vi "ORS_GalvoGenScanData3D_uw.vi"(0 "x_center":dbl, 1 "x_span":dbl=5.0, 2 "offset":dbl, 3 "span-factor":dbl=5.0, 4 "y_center":dbl, 5 "y_span":dbl=1.0, 6 "mode":i32=6, 7 "n_lines":i32=50, 8 "Custom trig.":T1={"n_frames to c. trig"=0, "custom trig length (frames)"=1, "n_frames between c. trig"=1, "n_custom trigger"=4}, 9 "n_frames same y pos":u32=4, 11 "flyback_lines":i32=4, 12 "galvo phase":i32, 13 "n_frames":i32=20, 16 "n_3D scans":u32=1 min=1, 17 "flyback frames":u16) -> (10 "t_data":dbl[](graph)=[5.0, 5.0, 5.0, 5.0, 5.0, 5.0, 5.0, 5.0, 5.0, 5.0, 5.0, 5.0, 5.0, 5.0, 5.0, 5.0, 5.0, 5.0, 5.0, 5.0, 5.0, 5.0, 5.0, 5.0, 5.0, 5.0, 5.0, 5.0, 5.0, 5.0, 5.0, 5.0, 5.0, 5.0, 5.0, 5.0, 5.0, 5.0, 5.0, 5.0, 5.0, 5.0, 5.0, 5.0, 5.0, 5.0, 5.0, 5.0, 5.0, 5.0, 0.0, 0.0, 0.0, 0.0, 5.0, 5.0, 5.0, 5.0, 5.0, 5.0, 5.0, 5.0, 5.0, 5.0, 5.0, 5.0, 5.0, 5.0, 5.0, 5.0, 5.0, 5.0, 5.0, 5.0, 5.0, 5.0, 5.0, 5.0, 5.0, 5.0, 5.0, 5.0, 5.0, 5.0, 5.0, 5.0, 5.0, 5.0, 5.0, 5.0, 5.0, 5.0, 5.0, 5.0, 5.0, 5.0, 5.0, 5.0, 5.0, 5.0, 5.0, 5.0, 5.0, 5.0, 0.0, 0.0, 0.0, 0.0, 5.0, 5.0, 5.0, 5.0, 5.0, 5.0, 5.0, 5.0, 5.0, 5.0, 5.0, 5.0, 5.0, 5.0, 5.0, 5.0, 5.0, 5.0, 5.0, 5.0, 5.0, 5.0, 5.0, 5.0, 5.0, 5.0, 5.0, 5.0, 5.0, 5.0, 5.0, 5.0, 5.0, 5.0, 5.0, 5.0, 5.0, 5.0, 5.0, 5.0, 5.0, 5.0, 5.0, 5.0, 5.0, 5.0, 5.0, 5.0, 5.0, 5.0, 0.0, 0.0, 0.0, 0.0, 5.0, 5.0, 5.0, 5.0, 5.0, 5.0, 5.0, 5.0, 5.0, 5.0, 5.0, 5.0, 5.0, 5.0, 5.0, 5.0, 5.0, 5.0, 5.0, 5.0, 5.0, 5.0, 5.0, 5.0, 5.0, 5.0, 5.0, 5.0, 5.0, 5.0, 5.0, 5.0, 5.0, 5.0, 5.0, 5.0, 5.0, 5.0, 5.0, 5.0, 5.0, 5.0, 5.0, 5.0, 5.0, 5.0, 5.0, 5.0, 5.0, 5.0, 0.0, 0.0, 0.0, 0.0, 5.0, 5.0, 5.0, 5.0, 5.0, 5.0, 5.0, 5.0, 5.0, 5.0, 5.0, 5.0, 5.0, 5.0, 5.0, 5.0, 5.0, 5.0, 5.0, 5.0, 5.0, 5.0, 5.0, 5.0, 5.0, 5.0, 5.0, 5.0, 5.0, 5.0, 5.0, 5.0, 5.0, 5.0, 5.0, 5.0, 5.0, 5.0, 5.0, 5.0, 5.0, 5.0, 5.0, 5.0, 5.0, 5.0, 5.0, 5.0, 5.0, 5.0, 0.0, 0.0, 0.0, 0.0, 5.0, 5.0, 5.0, 5.0, 5.0, 5.0, 5.0, 5.0, 5.0, 5.0, 5.0, 5.0, 5.0, 5.0, 5.0, 5.0, 5.0, 5.0, 5.0, 5.0, 5.0, 5.0, 5.0, 5.0, 5.0, 5.0, 5.0, 5.0, 5.0, 5.0, 5.0, 5.0, 5.0, 5.0, 5.0, 5.0, 5.0, 5.0, 5.0, 5.0, 5.0, 5.0, 5.0, 5.0, 5.0, 5.0, 5.0, 5.0, 5.0, 5.0, 0.0, 0.0, 0.0, 0.0, 5.0, 5.0, 5.0, 5.0, 5.0, 5.0, 5.0, 5.0, 5.0, 5.0, 5.0, 5.0, 5.0, 5.0, 5.0, 5.0, 5.0, 5.0, 5.0, 5.0, 5.0, 5.0, 5.0, 5.0, 5.0, 5.0, 5.0, 5.0, 5.0, 5.0, 5.0, 5.0, 5.0, 5.0, 5.0, 5.0, 5.0, 5.0, 5.0, 5.0, 5.0, 5.0, 5.0, 5.0, 5.0, 5.0, 5.0, 5.0, 5.0, 5.0, 0.0, 0.0, 0.0, 0.0, 5.0, 5.0, 5.0, 5.0, 5.0, 5.0, 5.0, 5.0, 5.0, 5.0, 5.0, 5.0, 5.0, 5.0, 5.0, 5.0, 5.0, 5.0, 5.0, 5.0, 5.0, 5.0, 5.0, 5.0, 5.0, 5.0, 5.0, 5.0, 5.0, 5.0, 5.0, 5.0, 5.0, 5.0, 5.0, 5.0, 5.0, 5.0, 5.0, 5.0, 5.0, 5.0, 5.0, 5.0, 5.0, 5.0, 5.0, 5.0, 5.0, 5.0, 0.0, 0.0, 0.0, 0.0, 5.0, 5.0, 5.0, 5.0, 5.0, 5.0, 5.0, 5.0, 5.0, 5.0, 5.0, 5.0, 5.0, 5.0, 5.0, 5.0, 5.0, 5.0, 5.0, 5.0, 5.0, 5.0, 5.0, 5.0, 5.0, 5.0, 5.0, 5.0, 5.0, 5.0, 5.0, 5.0, 5.0, 5.0, 5.0, 5.0, 5.0, 5.0, 5.0, 5.0, 5.0, 5.0, 5.0, 5.0, 5.0, 5.0, 5.0, 5.0, 5.0, 5.0, 0.0, 0.0, 0.0, 0.0, 5.0, 5.0, 5.0, 5.0, 5.0, 5.0, 5.0, 5.0, 5.0, 5.0, 5.0, 5.0, 5.0, 5.0, 5.0, 5.0, 5.0, 5.0, 5.0, 5.0, 5.0, 5.0, 5.0, 5.0, 5.0, 5.0, 5.0, 5.0, 5.0, 5.0, 5.0, 5.0, 5.0, 5.0, 5.0, 5.0, 5.0, 5.0, 5.0, 5.0, 5.0, 5.0, 5.0, 5.0, 5.0, 5.0, 5.0, 5.0, 5.0, 5.0, 0.0, 0.0, 0.0, 0.0, 5.0, 5.0, 5.0, 5.0, 5.0, 5.0, 5.0, 5.0, 5.0, 5.0, 5.0, 5.0, 5.0, 5.0, 5.0, 5.0, 5.0, 5.0, 5.0, 5.0, 5.0, 5.0, 5.0, 5.0, 5.0, 5.0, 5.0, 5.0, 5.0, 5.0, 5.0, 5.0, 5.0, 5.0, 5.0, 5.0, 5.0, 5.0, 5.0, 5.0, 5.0, 5.0, 5.0, 5.0, 5.0, 5.0, 5.0, 5.0, 5.0, 5.0, 0.0, 0.0, 0.0, 0.0, 5.0, 5.0, 5.0, 5.0, 5.0, 5.0, 5.0, 5.0, 5.0, 5.0, 5.0, 5.0, 5.0, 5.0, 5.0, 5.0, 5.0, 5.0, 5.0, 5.0, 5.0, 5.0, 5.0, 5.0, 5.0, 5.0, 5.0, 5.0, 5.0, 5.0, 5.0, 5.0, 5.0, 5.0, 5.0, 5.0, 5.0, 5.0, 5.0, 5.0, 5.0, 5.0, 5.0, 5.0, 5.0, 5.0, 5.0, 5.0, 5.0, 5.0, 0.0, 0.0, 0.0, 0.0, 5.0, 5.0, 5.0, 5.0, 5.0, 5.0, 5.0, 5.0, 5.0, 5.0, 5.0, 5.0, 5.0, 5.0, 5.0, 5.0, 5.0, 5.0, 5.0, 5.0, 5.0, 5.0, 5.0, 5.0, 5.0, 5.0, 5.0, 5.0, 5.0, 5.0, 5.0, 5.0, 5.0, 5.0, 5.0, 5.0, 5.0, 5.0, 5.0, 5.0, 5.0, 5.0, 5.0, 5.0, 5.0, 5.0, 5.0, 5.0, 5.0, 5.0, 0.0, 0.0, 0.0, 0.0, 5.0, 5.0, 5.0, 5.0, 5.0, 5.0, 5.0, 5.0, 5.0, 5.0, 5.0, 5.0, 5.0, 5.0, 5.0, 5.0, 5.0, 5.0, 5.0, 5.0, 5.0, 5.0, 5.0, 5.0, 5.0, 5.0, 5.0, 5.0, 5.0, 5.0, 5.0, 5.0, 5.0, 5.0, 5.0, 5.0, 5.0, 5.0, 5.0, 5.0, 5.0, 5.0, 5.0, 5.0, 5.0, 5.0, 5.0, 5.0, 5.0, 5.0, 0.0, 0.0, 0.0, 0.0, 5.0, 5.0, 5.0, 5.0, 5.0, 5.0, 5.0, 5.0, 5.0, 5.0, 5.0, 5.0, 5.0, 5.0, 5.0, 5.0, 5.0, 5.0, 5.0, 5.0, 5.0, 5.0, 5.0, 5.0, 5.0, 5.0, 5.0, 5.0, 5.0, 5.0, 5.0, 5.0, 5.0, 5.0, 5.0, 5.0, 5.0, 5.0, 5.0, 5.0, 5.0, 5.0, 5.0, 5.0, 5.0, 5.0, 5.0, 5.0, 5.0, 5.0, 0.0, 0.0, 0.0, 0.0, 5.0, 5.0, 5.0, 5.0, 5.0, 5.0, 5.0, 5.0, 5.0, 5.0, 5.0, 5.0, 5.0, 5.0, 5.0, 5.0, 5.0, 5.0, 5.0, 5.0, 5.0, 5.0, 5.0, 5.0, 5.0, 5.0, 5.0, 5.0, 5.0, 5.0, 5.0, 5.0, 5.0, 5.0, 5.0, 5.0, 5.0, 5.0, 5.0, 5.0, 5.0, 5.0, 5.0, 5.0, 5.0, 5.0, 5.0, 5.0, 5.0, 5.0, 0.0, 0.0, 0.0, 0.0, 5.0, 5.0, 5.0, 5.0, 5.0, 5.0, 5.0, 5.0, 5.0, 5.0, 5.0, 5.0, 5.0, 5.0, 5.0, 5.0, 5.0, 5.0, 5.0, 5.0, 5.0, 5.0, 5.0, 5.0, 5.0, 5.0, 5.0, 5.0, 5.0, 5.0, 5.0, 5.0, 5.0, 5.0, 5.0, 5.0, 5.0, 5.0, 5.0, 5.0, 5.0, 5.0, 5.0, 5.0, 5.0, 5.0, 5.0, 5.0, 5.0, 5.0, 0.0, 0.0, 0.0, 0.0, 5.0, 5.0, 5.0, 5.0, 5.0, 5.0, 5.0, 5.0, 5.0, 5.0, 5.0, 5.0, 5.0, 5.0, 5.0, 5.0, 5.0, 5.0, 5.0, 5.0, 5.0, 5.0, 5.0, 5.0, 5.0, 5.0, 5.0, 5.0, 5.0, 5.0, 5.0, 5.0, 5.0, 5.0, 5.0, 5.0, 5.0, 5.0, 5.0, 5.0, 5.0, 5.0, 5.0, 5.0, 5.0, 5.0, 5.0, 5.0, 5.0, 5.0, 0.0, 0.0, 0.0, 0.0, 5.0, 5.0, 5.0, 5.0, 5.0, 5.0, 5.0, 5.0, 5.0, 5.0, 5.0, 5.0, 5.0, 5.0, 5.0, 5.0, 5.0, 5.0, 5.0, 5.0, 5.0, 5.0, 5.0, 5.0, 5.0, 5.0, 5.0, 5.0, 5.0, 5.0, 5.0, 5.0, 5.0, 5.0, 5.0, 5.0, 5.0, 5.0, 5.0, 5.0, 5.0, 5.0, 5.0, 5.0, 5.0, 5.0, 5.0, 5.0, 5.0, 5.0, 0.0, 0.0, 0.0, 0.0, 5.0, 5.0, 5.0, 5.0, 5.0, 5.0, 5.0, 5.0, 5.0, 5.0, 5.0, 5.0, 5.0, 5.0, 5.0, 5.0, 5.0, 5.0, 5.0, 5.0, 5.0, 5.0, 5.0, 5.0, 5.0, 5.0, 5.0, 5.0, 5.0, 5.0, 5.0, 5.0, 5.0, 5.0, 5.0, 5.0, 5.0, 5.0, 5.0, 5.0, 5.0, 5.0, 5.0, 5.0, 5.0, 5.0, 5.0, 5.0, 5.0, 5.0, 0.0, 0.0, 0.0, 0.0], 14 "x_data":dbl[](graph)=[-2.5, -2.4, -2.3, -2.2, -2.1, -2.0, -1.9, -1.8, -1.7, -1.6, -1.5, -1.4, -1.3, -1.2, -1.1, -1.0, -0.8999999999999999, -0.8, -0.7, -0.6000000000000001, -0.5, -0.3999999999999999, -0.2999999999999998, -0.20000000000000018, -0.10000000000000009, 0.0, 0.10000000000000009, 0.20000000000000018, 0.2999999999999998, 0.3999999999999999, 0.5, 0.6000000000000001, 0.7000000000000002, 0.7999999999999998, 0.8999999999999999, 1.0, 1.1, 1.2000000000000002, 1.2999999999999998, 1.4, 1.5, 1.5999999999999996, 1.7000000000000002, 1.7999999999999998, 1.9000000000000004, 2.0, 2.0999999999999996, 2.2, 2.3, 2.4000000000000004, 2.5, 2.5, 0.0, -2.5, -2.5, -2.4, -2.3, -2.2, -2.1, -2.0, -1.9, -1.8, -1.7, -1.6, -1.5, -1.4, -1.3, -1.2, -1.1, -1.0, -0.8999999999999999, -0.8, -0.7, -0.6000000000000001, -0.5, -0.3999999999999999, -0.2999999999999998, -0.20000000000000018, -0.10000000000000009, 0.0, 0.10000000000000009, 0.20000000000000018, 0.2999999999999998, 0.3999999999999999, 0.5, 0.6000000000000001, 0.7000000000000002, 0.7999999999999998, 0.8999999999999999, 1.0, 1.1, 1.2000000000000002, 1.2999999999999998, 1.4, 1.5, 1.5999999999999996, 1.7000000000000002, 1.7999999999999998, 1.9000000000000004, 2.0, 2.0999999999999996, 2.2, 2.3, 2.4000000000000004, 2.5, 2.5, 0.0, -2.5, -2.5, -2.4, -2.3, -2.2, -2.1, -2.0, -1.9, -1.8, -1.7, -1.6, -1.5, -1.4, -1.3, -1.2, -1.1, -1.0, -0.8999999999999999, -0.8, -0.7, -0.6000000000000001, -0.5, -0.3999999999999999, -0.2999999999999998, -0.20000000000000018, -0.10000000000000009, 0.0, 0.10000000000000009, 0.20000000000000018, 0.2999999999999998, 0.3999999999999999, 0.5, 0.6000000000000001, 0.7000000000000002, 0.7999999999999998, 0.8999999999999999, 1.0, 1.1, 1.2000000000000002, 1.2999999999999998, 1.4, 1.5, 1.5999999999999996, 1.7000000000000002, 1.7999999999999998, 1.9000000000000004, 2.0, 2.0999999999999996, 2.2, 2.3, 2.4000000000000004, 2.5, 2.5, 0.0, -2.5, -2.5, -2.4, -2.3, -2.2, -2.1, -2.0, -1.9, -1.8, -1.7, -1.6, -1.5, -1.4, -1.3, -1.2, -1.1, -1.0, -0.8999999999999999, -0.8, -0.7, -0.6000000000000001, -0.5, -0.3999999999999999, -0.2999999999999998, -0.20000000000000018, -0.10000000000000009, 0.0, 0.10000000000000009, 0.20000000000000018, 0.2999999999999998, 0.3999999999999999, 0.5, 0.6000000000000001, 0.7000000000000002, 0.7999999999999998, 0.8999999999999999, 1.0, 1.1, 1.2000000000000002, 1.2999999999999998, 1.4, 1.5, 1.5999999999999996, 1.7000000000000002, 1.7999999999999998, 1.9000000000000004, 2.0, 2.0999999999999996, 2.2, 2.3, 2.4000000000000004, 2.5, 2.5, 0.0, -2.5, -2.5, -2.4, -2.3, -2.2, -2.1, -2.0, -1.9, -1.8, -1.7, -1.6, -1.5, -1.4, -1.3, -1.2, -1.1, -1.0, -0.8999999999999999, -0.8, -0.7, -0.6000000000000001, -0.5, -0.3999999999999999, -0.2999999999999998, -0.20000000000000018, -0.10000000000000009, 0.0, 0.10000000000000009, 0.20000000000000018, 0.2999999999999998, 0.3999999999999999, 0.5, 0.6000000000000001, 0.7000000000000002, 0.7999999999999998, 0.8999999999999999, 1.0, 1.1, 1.2000000000000002, 1.2999999999999998, 1.4, 1.5, 1.5999999999999996, 1.7000000000000002, 1.7999999999999998, 1.9000000000000004, 2.0, 2.0999999999999996, 2.2, 2.3, 2.4000000000000004, 2.5, 2.5, 0.0, -2.5, -2.5, -2.4, -2.3, -2.2, -2.1, -2.0, -1.9, -1.8, -1.7, -1.6, -1.5, -1.4, -1.3, -1.2, -1.1, -1.0, -0.8999999999999999, -0.8, -0.7, -0.6000000000000001, -0.5, -0.3999999999999999, -0.2999999999999998, -0.20000000000000018, -0.10000000000000009, 0.0, 0.10000000000000009, 0.20000000000000018, 0.2999999999999998, 0.3999999999999999, 0.5, 0.6000000000000001, 0.7000000000000002, 0.7999999999999998, 0.8999999999999999, 1.0, 1.1, 1.2000000000000002, 1.2999999999999998, 1.4, 1.5, 1.5999999999999996, 1.7000000000000002, 1.7999999999999998, 1.9000000000000004, 2.0, 2.0999999999999996, 2.2, 2.3, 2.4000000000000004, 2.5, 2.5, 0.0, -2.5, -2.5, -2.4, -2.3, -2.2, -2.1, -2.0, -1.9, -1.8, -1.7, -1.6, -1.5, -1.4, -1.3, -1.2, -1.1, -1.0, -0.8999999999999999, -0.8, -0.7, -0.6000000000000001, -0.5, -0.3999999999999999, -0.2999999999999998, -0.20000000000000018, -0.10000000000000009, 0.0, 0.10000000000000009, 0.20000000000000018, 0.2999999999999998, 0.3999999999999999, 0.5, 0.6000000000000001, 0.7000000000000002, 0.7999999999999998, 0.8999999999999999, 1.0, 1.1, 1.2000000000000002, 1.2999999999999998, 1.4, 1.5, 1.5999999999999996, 1.7000000000000002, 1.7999999999999998, 1.9000000000000004, 2.0, 2.0999999999999996, 2.2, 2.3, 2.4000000000000004, 2.5, 2.5, 0.0, -2.5, -2.5, -2.4, -2.3, -2.2, -2.1, -2.0, -1.9, -1.8, -1.7, -1.6, -1.5, -1.4, -1.3, -1.2, -1.1, -1.0, -0.8999999999999999, -0.8, -0.7, -0.6000000000000001, -0.5, -0.3999999999999999, -0.2999999999999998, -0.20000000000000018, -0.10000000000000009, 0.0, 0.10000000000000009, 0.20000000000000018, 0.2999999999999998, 0.3999999999999999, 0.5, 0.6000000000000001, 0.7000000000000002, 0.7999999999999998, 0.8999999999999999, 1.0, 1.1, 1.2000000000000002, 1.2999999999999998, 1.4, 1.5, 1.5999999999999996, 1.7000000000000002, 1.7999999999999998, 1.9000000000000004, 2.0, 2.0999999999999996, 2.2, 2.3, 2.4000000000000004, 2.5, 2.5, 0.0, -2.5, -2.5, -2.4, -2.3, -2.2, -2.1, -2.0, -1.9, -1.8, -1.7, -1.6, -1.5, -1.4, -1.3, -1.2, -1.1, -1.0, -0.8999999999999999, -0.8, -0.7, -0.6000000000000001, -0.5, -0.3999999999999999, -0.2999999999999998, -0.20000000000000018, -0.10000000000000009, 0.0, 0.10000000000000009, 0.20000000000000018, 0.2999999999999998, 0.3999999999999999, 0.5, 0.6000000000000001, 0.7000000000000002, 0.7999999999999998, 0.8999999999999999, 1.0, 1.1, 1.2000000000000002, 1.2999999999999998, 1.4, 1.5, 1.5999999999999996, 1.7000000000000002, 1.7999999999999998, 1.9000000000000004, 2.0, 2.0999999999999996, 2.2, 2.3, 2.4000000000000004, 2.5, 2.5, 0.0, -2.5, -2.5, -2.4, -2.3, -2.2, -2.1, -2.0, -1.9, -1.8, -1.7, -1.6, -1.5, -1.4, -1.3, -1.2, -1.1, -1.0, -0.8999999999999999, -0.8, -0.7, -0.6000000000000001, -0.5, -0.3999999999999999, -0.2999999999999998, -0.20000000000000018, -0.10000000000000009, 0.0, 0.10000000000000009, 0.20000000000000018, 0.2999999999999998, 0.3999999999999999, 0.5, 0.6000000000000001, 0.7000000000000002, 0.7999999999999998, 0.8999999999999999, 1.0, 1.1, 1.2000000000000002, 1.2999999999999998, 1.4, 1.5, 1.5999999999999996, 1.7000000000000002, 1.7999999999999998, 1.9000000000000004, 2.0, 2.0999999999999996, 2.2, 2.3, 2.4000000000000004, 2.5, 2.5, 0.0, -2.5, -2.5, -2.4, -2.3, -2.2, -2.1, -2.0, -1.9, -1.8, -1.7, -1.6, -1.5, -1.4, -1.3, -1.2, -1.1, -1.0, -0.8999999999999999, -0.8, -0.7, -0.6000000000000001, -0.5, -0.3999999999999999, -0.2999999999999998, -0.20000000000000018, -0.10000000000000009, 0.0, 0.10000000000000009, 0.20000000000000018, 0.2999999999999998, 0.3999999999999999, 0.5, 0.6000000000000001, 0.7000000000000002, 0.7999999999999998, 0.8999999999999999, 1.0, 1.1, 1.2000000000000002, 1.2999999999999998, 1.4, 1.5, 1.5999999999999996, 1.7000000000000002, 1.7999999999999998, 1.9000000000000004, 2.0, 2.0999999999999996, 2.2, 2.3, 2.4000000000000004, 2.5, 2.5, 0.0, -2.5, -2.5, -2.4, -2.3, -2.2, -2.1, -2.0, -1.9, -1.8, -1.7, -1.6, -1.5, -1.4, -1.3, -1.2, -1.1, -1.0, -0.8999999999999999, -0.8, -0.7, -0.6000000000000001, -0.5, -0.3999999999999999, -0.2999999999999998, -0.20000000000000018, -0.10000000000000009, 0.0, 0.10000000000000009, 0.20000000000000018, 0.2999999999999998, 0.3999999999999999, 0.5, 0.6000000000000001, 0.7000000000000002, 0.7999999999999998, 0.8999999999999999, 1.0, 1.1, 1.2000000000000002, 1.2999999999999998, 1.4, 1.5, 1.5999999999999996, 1.7000000000000002, 1.7999999999999998, 1.9000000000000004, 2.0, 2.0999999999999996, 2.2, 2.3, 2.4000000000000004, 2.5, 2.5, 0.0, -2.5, -2.5, -2.4, -2.3, -2.2, -2.1, -2.0, -1.9, -1.8, -1.7, -1.6, -1.5, -1.4, -1.3, -1.2, -1.1, -1.0, -0.8999999999999999, -0.8, -0.7, -0.6000000000000001, -0.5, -0.3999999999999999, -0.2999999999999998, -0.20000000000000018, -0.10000000000000009, 0.0, 0.10000000000000009, 0.20000000000000018, 0.2999999999999998, 0.3999999999999999, 0.5, 0.6000000000000001, 0.7000000000000002, 0.7999999999999998, 0.8999999999999999, 1.0, 1.1, 1.2000000000000002, 1.2999999999999998, 1.4, 1.5, 1.5999999999999996, 1.7000000000000002, 1.7999999999999998, 1.9000000000000004, 2.0, 2.0999999999999996, 2.2, 2.3, 2.4000000000000004, 2.5, 2.5, 0.0, -2.5, -2.5, -2.4, -2.3, -2.2, -2.1, -2.0, -1.9, -1.8, -1.7, -1.6, -1.5, -1.4, -1.3, -1.2, -1.1, -1.0, -0.8999999999999999, -0.8, -0.7, -0.6000000000000001, -0.5, -0.3999999999999999, -0.2999999999999998, -0.20000000000000018, -0.10000000000000009, 0.0, 0.10000000000000009, 0.20000000000000018, 0.2999999999999998, 0.3999999999999999, 0.5, 0.6000000000000001, 0.7000000000000002, 0.7999999999999998, 0.8999999999999999, 1.0, 1.1, 1.2000000000000002, 1.2999999999999998, 1.4, 1.5, 1.5999999999999996, 1.7000000000000002, 1.7999999999999998, 1.9000000000000004, 2.0, 2.0999999999999996, 2.2, 2.3, 2.4000000000000004, 2.5, 2.5, 0.0, -2.5, -2.5, -2.4, -2.3, -2.2, -2.1, -2.0, -1.9, -1.8, -1.7, -1.6, -1.5, -1.4, -1.3, -1.2, -1.1, -1.0, -0.8999999999999999, -0.8, -0.7, -0.6000000000000001, -0.5, -0.3999999999999999, -0.2999999999999998, -0.20000000000000018, -0.10000000000000009, 0.0, 0.10000000000000009, 0.20000000000000018, 0.2999999999999998, 0.3999999999999999, 0.5, 0.6000000000000001, 0.7000000000000002, 0.7999999999999998, 0.8999999999999999, 1.0, 1.1, 1.2000000000000002, 1.2999999999999998, 1.4, 1.5, 1.5999999999999996, 1.7000000000000002, 1.7999999999999998, 1.9000000000000004, 2.0, 2.0999999999999996, 2.2, 2.3, 2.4000000000000004, 2.5, 2.5, 0.0, -2.5, -2.5, -2.4, -2.3, -2.2, -2.1, -2.0, -1.9, -1.8, -1.7, -1.6, -1.5, -1.4, -1.3, -1.2, -1.1, -1.0, -0.8999999999999999, -0.8, -0.7, -0.6000000000000001, -0.5, -0.3999999999999999, -0.2999999999999998, -0.20000000000000018, -0.10000000000000009, 0.0, 0.10000000000000009, 0.20000000000000018, 0.2999999999999998, 0.3999999999999999, 0.5, 0.6000000000000001, 0.7000000000000002, 0.7999999999999998, 0.8999999999999999, 1.0, 1.1, 1.2000000000000002, 1.2999999999999998, 1.4, 1.5, 1.5999999999999996, 1.7000000000000002, 1.7999999999999998, 1.9000000000000004, 2.0, 2.0999999999999996, 2.2, 2.3, 2.4000000000000004, 2.5, 2.5, 0.0, -2.5, -2.5, -2.4, -2.3, -2.2, -2.1, -2.0, -1.9, -1.8, -1.7, -1.6, -1.5, -1.4, -1.3, -1.2, -1.1, -1.0, -0.8999999999999999, -0.8, -0.7, -0.6000000000000001, -0.5, -0.3999999999999999, -0.2999999999999998, -0.20000000000000018, -0.10000000000000009, 0.0, 0.10000000000000009, 0.20000000000000018, 0.2999999999999998, 0.3999999999999999, 0.5, 0.6000000000000001, 0.7000000000000002, 0.7999999999999998, 0.8999999999999999, 1.0, 1.1, 1.2000000000000002, 1.2999999999999998, 1.4, 1.5, 1.5999999999999996, 1.7000000000000002, 1.7999999999999998, 1.9000000000000004, 2.0, 2.0999999999999996, 2.2, 2.3, 2.4000000000000004, 2.5, 2.5, 0.0, -2.5, -2.5, -2.4, -2.3, -2.2, -2.1, -2.0, -1.9, -1.8, -1.7, -1.6, -1.5, -1.4, -1.3, -1.2, -1.1, -1.0, -0.8999999999999999, -0.8, -0.7, -0.6000000000000001, -0.5, -0.3999999999999999, -0.2999999999999998, -0.20000000000000018, -0.10000000000000009, 0.0, 0.10000000000000009, 0.20000000000000018, 0.2999999999999998, 0.3999999999999999, 0.5, 0.6000000000000001, 0.7000000000000002, 0.7999999999999998, 0.8999999999999999, 1.0, 1.1, 1.2000000000000002, 1.2999999999999998, 1.4, 1.5, 1.5999999999999996, 1.7000000000000002, 1.7999999999999998, 1.9000000000000004, 2.0, 2.0999999999999996, 2.2, 2.3, 2.4000000000000004, 2.5, 2.5, 0.0, -2.5, -2.5, -2.4, -2.3, -2.2, -2.1, -2.0, -1.9, -1.8, -1.7, -1.6, -1.5, -1.4, -1.3, -1.2, -1.1, -1.0, -0.8999999999999999, -0.8, -0.7, -0.6000000000000001, -0.5, -0.3999999999999999, -0.2999999999999998, -0.20000000000000018, -0.10000000000000009, 0.0, 0.10000000000000009, 0.20000000000000018, 0.2999999999999998, 0.3999999999999999, 0.5, 0.6000000000000001, 0.7000000000000002, 0.7999999999999998, 0.8999999999999999, 1.0, 1.1, 1.2000000000000002, 1.2999999999999998, 1.4, 1.5, 1.5999999999999996, 1.7000000000000002, 1.7999999999999998, 1.9000000000000004, 2.0, 2.0999999999999996, 2.2, 2.3, 2.4000000000000004, 2.5, 2.5, 0.0, -2.5, -2.5, -2.4, -2.3, -2.2, -2.1, -2.0, -1.9, -1.8, -1.7, -1.6, -1.5, -1.4, -1.3, -1.2, -1.1, -1.0, -0.8999999999999999, -0.8, -0.7, -0.6000000000000001, -0.5, -0.3999999999999999, -0.2999999999999998, -0.20000000000000018, -0.10000000000000009, 0.0, 0.10000000000000009, 0.20000000000000018, 0.2999999999999998, 0.3999999999999999, 0.5, 0.6000000000000001, 0.7000000000000002, 0.7999999999999998, 0.8999999999999999, 1.0, 1.1, 1.2000000000000002, 1.2999999999999998, 1.4, 1.5, 1.5999999999999996, 1.7000000000000002, 1.7999999999999998, 1.9000000000000004, 2.0, 2.0999999999999996, 2.2, 2.3, 2.4000000000000004, 2.5, 2.5, 0.0, -2.5], 15 "y_data":dbl[](graph)=[-0.5, -0.5, -0.5, -0.5, -0.5, -0.5, -0.5, -0.5, -0.5, -0.5, -0.5, -0.5, -0.5, -0.5, -0.5, -0.5, -0.5, -0.5, -0.5, -0.5, -0.5, -0.5, -0.5, -0.5, -0.5, -0.5, -0.5, -0.5, -0.5, -0.5, -0.5, -0.5, -0.5, -0.5, -0.5, -0.5, -0.5, -0.5, -0.5, -0.5, -0.5, -0.5, -0.5, -0.5, -0.5, -0.5, -0.5, -0.5, -0.5, -0.5, -0.5, -0.5, -0.5, -0.5, -0.5, -0.5, -0.5, -0.5, -0.5, -0.5, -0.5, -0.5, -0.5, -0.5, -0.5, -0.5, -0.5, -0.5, -0.5, -0.5, -0.5, -0.5, -0.5, -0.5, -0.5, -0.5, -0.5, -0.5, -0.5, -0.5, -0.5, -0.5, -0.5, -0.5, -0.5, -0.5, -0.5, -0.5, -0.5, -0.5, -0.5, -0.5, -0.5, -0.5, -0.5, -0.5, -0.5, -0.5, -0.5, -0.5, -0.5, -0.5, -0.5, -0.5, -0.5, -0.5, -0.5, -0.5, -0.5, -0.5, -0.5, -0.5, -0.5, -0.5, -0.5, -0.5, -0.5, -0.5, -0.5, -0.5, -0.5, -0.5, -0.5, -0.5, -0.5, -0.5, -0.5, -0.5, -0.5, -0.5, -0.5, -0.5, -0.5, -0.5, -0.5, -0.5, -0.5, -0.5, -0.5, -0.5, -0.5, -0.5, -0.5, -0.5, -0.5, -0.5, -0.5, -0.5, -0.5, -0.5, -0.5, -0.5, -0.5, -0.5, -0.5, -0.5, -0.5, -0.5, -0.5, -0.5, -0.5, -0.5, -0.5, -0.5, -0.5, -0.5, -0.5, -0.5, -0.5, -0.5, -0.5, -0.5, -0.5, -0.5, -0.5, -0.5, -0.5, -0.5, -0.5, -0.5, -0.5, -0.5, -0.5, -0.5, -0.5, -0.5, -0.5, -0.5, -0.5, -0.5, -0.5, -0.5, -0.5, -0.5, -0.5, -0.5, -0.5, -0.5, -0.5, -0.5, -0.5, -0.5, -0.5, -0.5, -0.5, -0.5, -0.5, -0.5, -0.5, -0.5, -0.5, -0.5, -0.5, -0.25, -0.25, -0.25, -0.25, -0.25, -0.25, -0.25, -0.25, -0.25, -0.25, -0.25, -0.25, -0.25, -0.25, -0.25, -0.25, -0.25, -0.25, -0.25, -0.25, -0.25, -0.25, -0.25, -0.25, -0.25, -0.25, -0.25, -0.25, -0.25, -0.25, -0.25, -0.25, -0.25, -0.25, -0.25, -0.25, -0.25, -0.25, -0.25, -0.25, -0.25, -0.25, -0.25, -0.25, -0.25, -0.25, -0.25, -0.25, -0.25, -0.25, -0.25, -0.25, -0.25, -0.25, -0.25, -0.25, -0.25, -0.25, -0.25, -0.25, -0.25, -0.25, -0.25, -0.25, -0.25, -0.25, -0.25, -0.25, -0.25, -0.25, -0.25, -0.25, -0.25, -0.25, -0.25, -0.25, -0.25, -0.25, -0.25, -0.25, -0.25, -0.25, -0.25, -0.25, -0.25, -0.25, -0.25, -0.25, -0.25, -0.25, -0.25, -0.25, -0.25, -0.25, -0.25, -0.25, -0.25, -0.25, -0.25, -0.25, -0.25, -0.25, -0.25, -0.25, -0.25, -0.25, -0.25, -0.25, -0.25, -0.25, -0.25, -0.25, -0.25, -0.25, -0.25, -0.25, -0.25, -0.25, -0.25, -0.25, -0.25, -0.25, -0.25, -0.25, -0.25, -0.25, -0.25, -0.25, -0.25, -0.25, -0.25, -0.25, -0.25, -0.25, -0.25, -0.25, -0.25, -0.25, -0.25, -0.25, -0.25, -0.25, -0.25, -0.25, -0.25, -0.25, -0.25, -0.25, -0.25, -0.25, -0.25, -0.25, -0.25, -0.25, -0.25, -0.25, -0.25, -0.25, -0.25, -0.25, -0.25, -0.25, -0.25, -0.25, -0.25, -0.25, -0.25, -0.25, -0.25, -0.25, -0.25, -0.25, -0.25, -0.25, -0.25, -0.25, -0.25, -0.25, -0.25, -0.25, -0.25, -0.25, -0.25, -0.25, -0.25, -0.25, -0.25, -0.25, -0.25, -0.25, -0.25, -0.25, -0.25, -0.25, -0.25, -0.25, -0.25, -0.25, -0.25, -0.25, -0.25, -0.25, -0.25, -0.25, -0.25, -0.25, -0.25, -0.25, -0.25, -0.25, -0.25, -0.25, -0.25, -0.25, -0.25, -0.25, 0.0, 0.0, 0.0, 0.0, 0.0, 0.0, 0.0, 0.0, 0.0, 0.0, 0.0, 0.0, 0.0, 0.0, 0.0, 0.0, 0.0, 0.0, 0.0, 0.0, 0.0, 0.0, 0.0, 0.0, 0.0, 0.0, 0.0, 0.0, 0.0, 0.0, 0.0, 0.0, 0.0, 0.0, 0.0, 0.0, 0.0, 0.0, 0.0, 0.0, 0.0, 0.0, 0.0, 0.0, 0.0, 0.0, 0.0, 0.0, 0.0, 0.0, 0.0, 0.0, 0.0, 0.0, 0.0, 0.0, 0.0, 0.0, 0.0, 0.0, 0.0, 0.0, 0.0, 0.0, 0.0, 0.0, 0.0, 0.0, 0.0, 0.0, 0.0, 0.0, 0.0, 0.0, 0.0, 0.0, 0.0, 0.0, 0.0, 0.0, 0.0, 0.0, 0.0, 0.0, 0.0, 0.0, 0.0, 0.0, 0.0, 0.0, 0.0, 0.0, 0.0, 0.0, 0.0, 0.0, 0.0, 0.0, 0.0, 0.0, 0.0, 0.0, 0.0, 0.0, 0.0, 0.0, 0.0, 0.0, 0.0, 0.0, 0.0, 0.0, 0.0, 0.0, 0.0, 0.0, 0.0, 0.0, 0.0, 0.0, 0.0, 0.0, 0.0, 0.0, 0.0, 0.0, 0.0, 0.0, 0.0, 0.0, 0.0, 0.0, 0.0, 0.0, 0.0, 0.0, 0.0, 0.0, 0.0, 0.0, 0.0, 0.0, 0.0, 0.0, 0.0, 0.0, 0.0, 0.0, 0.0, 0.0, 0.0, 0.0, 0.0, 0.0, 0.0, 0.0, 0.0, 0.0, 0.0, 0.0, 0.0, 0.0, 0.0, 0.0, 0.0, 0.0, 0.0, 0.0, 0.0, 0.0, 0.0, 0.0, 0.0, 0.0, 0.0, 0.0, 0.0, 0.0, 0.0, 0.0, 0.0, 0.0, 0.0, 0.0, 0.0, 0.0, 0.0, 0.0, 0.0, 0.0, 0.0, 0.0, 0.0, 0.0, 0.0, 0.0, 0.0, 0.0, 0.0, 0.0, 0.0, 0.0, 0.0, 0.0, 0.0, 0.0, 0.0, 0.0, 0.0, 0.0, 0.0, 0.0, 0.0, 0.0, 0.0, 0.0, 0.25, 0.25, 0.25, 0.25, 0.25, 0.25, 0.25, 0.25, 0.25, 0.25, 0.25, 0.25, 0.25, 0.25, 0.25, 0.25, 0.25, 0.25, 0.25, 0.25, 0.25, 0.25, 0.25, 0.25, 0.25, 0.25, 0.25, 0.25, 0.25, 0.25, 0.25, 0.25, 0.25, 0.25, 0.25, 0.25, 0.25, 0.25, 0.25, 0.25, 0.25, 0.25, 0.25, 0.25, 0.25, 0.25, 0.25, 0.25, 0.25, 0.25, 0.25, 0.25, 0.25, 0.25, 0.25, 0.25, 0.25, 0.25, 0.25, 0.25, 0.25, 0.25, 0.25, 0.25, 0.25, 0.25, 0.25, 0.25, 0.25, 0.25, 0.25, 0.25, 0.25, 0.25, 0.25, 0.25, 0.25, 0.25, 0.25, 0.25, 0.25, 0.25, 0.25, 0.25, 0.25, 0.25, 0.25, 0.25, 0.25, 0.25, 0.25, 0.25, 0.25, 0.25, 0.25, 0.25, 0.25, 0.25, 0.25, 0.25, 0.25, 0.25, 0.25, 0.25, 0.25, 0.25, 0.25, 0.25, 0.25, 0.25, 0.25, 0.25, 0.25, 0.25, 0.25, 0.25, 0.25, 0.25, 0.25, 0.25, 0.25, 0.25, 0.25, 0.25, 0.25, 0.25, 0.25, 0.25, 0.25, 0.25, 0.25, 0.25, 0.25, 0.25, 0.25, 0.25, 0.25, 0.25, 0.25, 0.25, 0.25, 0.25, 0.25, 0.25, 0.25, 0.25, 0.25, 0.25, 0.25, 0.25, 0.25, 0.25, 0.25, 0.25, 0.25, 0.25, 0.25, 0.25, 0.25, 0.25, 0.25, 0.25, 0.25, 0.25, 0.25, 0.25, 0.25, 0.25, 0.25, 0.25, 0.25, 0.25, 0.25, 0.25, 0.25, 0.25, 0.25, 0.25, 0.25, 0.25, 0.25, 0.25, 0.25, 0.25, 0.25, 0.25, 0.25, 0.25, 0.25, 0.25, 0.25, 0.25, 0.25, 0.25, 0.25, 0.25, 0.25, 0.25, 0.25, 0.25, 0.25, 0.25, 0.25, 0.25, 0.25, 0.25, 0.25, 0.25, 0.25, 0.25, 0.25, 0.25, 0.25, 0.25, 0.25, 0.25, 0.5, 0.5, 0.5, 0.5, 0.5, 0.5, 0.5, 0.5, 0.5, 0.5, 0.5, 0.5, 0.5, 0.5, 0.5, 0.5, 0.5, 0.5, 0.5, 0.5, 0.5, 0.5, 0.5, 0.5, 0.5, 0.5, 0.5, 0.5, 0.5, 0.5, 0.5, 0.5, 0.5, 0.5, 0.5, 0.5, 0.5, 0.5, 0.5, 0.5, 0.5, 0.5, 0.5, 0.5, 0.5, 0.5, 0.5, 0.5, 0.5, 0.5, 0.5, 0.5, 0.5, 0.5, 0.5, 0.5, 0.5, 0.5, 0.5, 0.5, 0.5, 0.5, 0.5, 0.5, 0.5, 0.5, 0.5, 0.5, 0.5, 0.5, 0.5, 0.5, 0.5, 0.5, 0.5, 0.5, 0.5, 0.5, 0.5, 0.5, 0.5, 0.5, 0.5, 0.5, 0.5, 0.5, 0.5, 0.5, 0.5, 0.5, 0.5, 0.5, 0.5, 0.5, 0.5, 0.5, 0.5, 0.5, 0.5, 0.5, 0.5, 0.5, 0.5, 0.5, 0.5, 0.5, 0.5, 0.5, 0.5, 0.5, 0.5, 0.5, 0.5, 0.5, 0.5, 0.5, 0.5, 0.5, 0.5, 0.5, 0.5, 0.5, 0.5, 0.5, 0.5, 0.5, 0.5, 0.5, 0.5, 0.5, 0.5, 0.5, 0.5, 0.5, 0.5, 0.5, 0.5, 0.5, 0.5, 0.5, 0.5, 0.5, 0.5, 0.5, 0.5, 0.5, 0.5, 0.5, 0.5, 0.5, 0.5, 0.5, 0.5, 0.5, 0.5, 0.5, 0.5, 0.5, 0.5, 0.5, 0.5, 0.5, 0.5, 0.5, 0.5, 0.5, 0.5, 0.5, 0.5, 0.5, 0.5, 0.5, 0.5, 0.5, 0.5, 0.5, 0.5, 0.5, 0.5, 0.5, 0.5, 0.5, 0.5, 0.5, 0.5, 0.5, 0.5, 0.5, 0.5, 0.5, 0.5, 0.5, 0.5, 0.5, 0.5, 0.5, 0.5, 0.5, 0.5, 0.5, 0.5, 0.5, 0.5, 0.5, 0.5, 0.5, 0.5, 0.5, 0.5, 0.5, 0.5, 0.5, 0.5, 0.5, 0.5, 0.5, -0.5, -0.5, -0.5], 18 "trigger out":u32[](graph)=[4294967295, 4294967295, 4294967295, 4294967295, 4294967295, 4294967295, 4294967295, 4294967295, 4294967295, 4294967295, 4294967295, 4294967295, 4294967295, 4294967295, 4294967295, 4294967295, 4294967295, 4294967295, 4294967295, 4294967295, 4294967295, 4294967295, 4294967295, 4294967295, 4294967295, 4294967295, 4294967295, 4294967295, 4294967295, 4294967295, 4294967295, 4294967295, 4294967295, 4294967295, 4294967295, 4294967295, 4294967295, 4294967295, 4294967295, 4294967295, 4294967295, 4294967295, 4294967295, 4294967295, 4294967295, 4294967295, 4294967295, 4294967295, 4294967295, 4294967295, 0, 0, 0, 0, 4294967295, 4294967295, 4294967295, 4294967295, 4294967295, 4294967295, 4294967295, 4294967295, 4294967295, 4294967295, 4294967295, 4294967295, 4294967295, 4294967295, 4294967295, 4294967295, 4294967295, 4294967295, 4294967295, 4294967295, 4294967295, 4294967295, 4294967295, 4294967295, 4294967295, 4294967295, 4294967295, 4294967295, 4294967295, 4294967295, 4294967295, 4294967295, 4294967295, 4294967295, 4294967295, 4294967295, 4294967295, 4294967295, 4294967295, 4294967295, 4294967295, 4294967295, 4294967295, 4294967295, 4294967295, 4294967295, 4294967295, 4294967295, 4294967295, 4294967295, 0, 0, 0, 0, 4294967295, 4294967295, 4294967295, 4294967295, 4294967295, 4294967295, 4294967295, 4294967295, 4294967295, 4294967295, 4294967295, 4294967295, 4294967295, 4294967295, 4294967295, 4294967295, 4294967295, 4294967295, 4294967295, 4294967295, 4294967295, 4294967295, 4294967295, 4294967295, 4294967295, 4294967295, 4294967295, 4294967295, 4294967295, 4294967295, 4294967295, 4294967295, 4294967295, 4294967295, 4294967295, 4294967295, 4294967295, 4294967295, 4294967295, 4294967295, 4294967295, 4294967295, 4294967295, 4294967295, 4294967295, 4294967295, 4294967295, 4294967295, 4294967295, 4294967295, 0, 0, 0, 0, 4294967295, 4294967295, 4294967295, 4294967295, 4294967295, 4294967295, 4294967295, 4294967295, 4294967295, 4294967295, 4294967295, 4294967295, 4294967295, 4294967295, 4294967295, 4294967295, 4294967295, 4294967295, 4294967295, 4294967295, 4294967295, 4294967295, 4294967295, 4294967295, 4294967295, 4294967295, 4294967295, 4294967295, 4294967295, 4294967295, 4294967295, 4294967295, 4294967295, 4294967295, 4294967295, 4294967295, 4294967295, 4294967295, 4294967295, 4294967295, 4294967295, 4294967295, 4294967295, 4294967295, 4294967295, 4294967295, 4294967295, 4294967295, 4294967295, 4294967295, 0, 0, 0, 0, 4294967295, 4294967295, 4294967295, 4294967295, 4294967295, 4294967295, 4294967295, 4294967295, 4294967295, 4294967295, 4294967295, 4294967295, 4294967295, 4294967295, 4294967295, 4294967295, 4294967295, 4294967295, 4294967295, 4294967295, 4294967295, 4294967295, 4294967295, 4294967295, 4294967295, 4294967295, 4294967295, 4294967295, 4294967295, 4294967295, 4294967295, 4294967295, 4294967295, 4294967295, 4294967295, 4294967295, 4294967295, 4294967295, 4294967295, 4294967295, 4294967295, 4294967295, 4294967295, 4294967295, 4294967295, 4294967295, 4294967295, 4294967295, 4294967295, 4294967295, 0, 0, 0, 0, 4294967295, 4294967295, 4294967295, 4294967295, 4294967295, 4294967295, 4294967295, 4294967295, 4294967295, 4294967295, 4294967295, 4294967295, 4294967295, 4294967295, 4294967295, 4294967295, 4294967295, 4294967295, 4294967295, 4294967295, 4294967295, 4294967295, 4294967295, 4294967295, 4294967295, 4294967295, 4294967295, 4294967295, 4294967295, 4294967295, 4294967295, 4294967295, 4294967295, 4294967295, 4294967295, 4294967295, 4294967295, 4294967295, 4294967295, 4294967295, 4294967295, 4294967295, 4294967295, 4294967295, 4294967295, 4294967295, 4294967295, 4294967295, 4294967295, 4294967295, 0, 0, 0, 0, 4294967295, 4294967295, 4294967295, 4294967295, 4294967295, 4294967295, 4294967295, 4294967295, 4294967295, 4294967295, 4294967295, 4294967295, 4294967295, 4294967295, 4294967295, 4294967295, 4294967295, 4294967295, 4294967295, 4294967295, 4294967295, 4294967295, 4294967295, 4294967295, 4294967295, 4294967295, 4294967295, 4294967295, 4294967295, 4294967295, 4294967295, 4294967295, 4294967295, 4294967295, 4294967295, 4294967295, 4294967295, 4294967295, 4294967295, 4294967295, 4294967295, 4294967295, 4294967295, 4294967295, 4294967295, 4294967295, 4294967295, 4294967295, 4294967295, 4294967295, 0, 0, 0, 0, 4294967295, 4294967295, 4294967295, 4294967295, 4294967295, 4294967295, 4294967295, 4294967295, 4294967295, 4294967295, 4294967295, 4294967295, 4294967295, 4294967295, 4294967295, 4294967295, 4294967295, 4294967295, 4294967295, 4294967295, 4294967295, 4294967295, 4294967295, 4294967295, 4294967295, 4294967295, 4294967295, 4294967295, 4294967295, 4294967295, 4294967295, 4294967295, 4294967295, 4294967295, 4294967295, 4294967295, 4294967295, 4294967295, 4294967295, 4294967295, 4294967295, 4294967295, 4294967295, 4294967295, 4294967295, 4294967295, 4294967295, 4294967295, 4294967295, 4294967295, 0, 0, 0, 0, 4294967295, 4294967295, 4294967295, 4294967295, 4294967295, 4294967295, 4294967295, 4294967295, 4294967295, 4294967295, 4294967295, 4294967295, 4294967295, 4294967295, 4294967295, 4294967295, 4294967295, 4294967295, 4294967295, 4294967295, 4294967295, 4294967295, 4294967295, 4294967295, 4294967295, 4294967295, 4294967295, 4294967295, 4294967295, 4294967295, 4294967295, 4294967295, 4294967295, 4294967295, 4294967295, 4294967295, 4294967295, 4294967295, 4294967295, 4294967295, 4294967295, 4294967295, 4294967295, 4294967295, 4294967295, 4294967295, 4294967295, 4294967295, 4294967295, 4294967295, 0, 0, 0, 0, 4294967295, 4294967295, 4294967295, 4294967295, 4294967295, 4294967295, 4294967295, 4294967295, 4294967295, 4294967295, 4294967295, 4294967295, 4294967295, 4294967295, 4294967295, 4294967295, 4294967295, 4294967295, 4294967295, 4294967295, 4294967295, 4294967295, 4294967295, 4294967295, 4294967295, 4294967295, 4294967295, 4294967295, 4294967295, 4294967295, 4294967295, 4294967295, 4294967295, 4294967295, 4294967295, 4294967295, 4294967295, 4294967295, 4294967295, 4294967295, 4294967295, 4294967295, 4294967295, 4294967295, 4294967295, 4294967295, 4294967295, 4294967295, 4294967295, 4294967295, 0, 0, 0, 0, 4294967295, 4294967295, 4294967295, 4294967295, 4294967295, 4294967295, 4294967295, 4294967295, 4294967295, 4294967295, 4294967295, 4294967295, 4294967295, 4294967295, 4294967295, 4294967295, 4294967295, 4294967295, 4294967295, 4294967295, 4294967295, 4294967295, 4294967295, 4294967295, 4294967295, 4294967295, 4294967295, 4294967295, 4294967295, 4294967295, 4294967295, 4294967295, 4294967295, 4294967295, 4294967295, 4294967295, 4294967295, 4294967295, 4294967295, 4294967295, 4294967295, 4294967295, 4294967295, 4294967295, 4294967295, 4294967295, 4294967295, 4294967295, 4294967295, 4294967295, 0, 0, 0, 0, 4294967295, 4294967295, 4294967295, 4294967295, 4294967295, 4294967295, 4294967295, 4294967295, 4294967295, 4294967295, 4294967295, 4294967295, 4294967295, 4294967295, 4294967295, 4294967295, 4294967295, 4294967295, 4294967295, 4294967295, 4294967295, 4294967295, 4294967295, 4294967295, 4294967295, 4294967295, 4294967295, 4294967295, 4294967295, 4294967295, 4294967295, 4294967295, 4294967295, 4294967295, 4294967295, 4294967295, 4294967295, 4294967295, 4294967295, 4294967295, 4294967295, 4294967295, 4294967295, 4294967295, 4294967295, 4294967295, 4294967295, 4294967295, 4294967295, 4294967295, 0, 0, 0, 0, 4294967295, 4294967295, 4294967295, 4294967295, 4294967295, 4294967295, 4294967295, 4294967295, 4294967295, 4294967295, 4294967295, 4294967295, 4294967295, 4294967295, 4294967295, 4294967295, 4294967295, 4294967295, 4294967295, 4294967295, 4294967295, 4294967295, 4294967295, 4294967295, 4294967295, 4294967295, 4294967295, 4294967295, 4294967295, 4294967295, 4294967295, 4294967295, 4294967295, 4294967295, 4294967295, 4294967295, 4294967295, 4294967295, 4294967295, 4294967295, 4294967295, 4294967295, 4294967295, 4294967295, 4294967295, 4294967295, 4294967295, 4294967295, 4294967295, 4294967295, 0, 0, 0, 0, 4294967295, 4294967295, 4294967295, 4294967295, 4294967295, 4294967295, 4294967295, 4294967295, 4294967295, 4294967295, 4294967295, 4294967295, 4294967295, 4294967295, 4294967295, 4294967295, 4294967295, 4294967295, 4294967295, 4294967295, 4294967295, 4294967295, 4294967295, 4294967295, 4294967295, 4294967295, 4294967295, 4294967295, 4294967295, 4294967295, 4294967295, 4294967295, 4294967295, 4294967295, 4294967295, 4294967295, 4294967295, 4294967295, 4294967295, 4294967295, 4294967295, 4294967295, 4294967295, 4294967295, 4294967295, 4294967295, 4294967295, 4294967295, 4294967295, 4294967295, 0, 0, 0, 0, 4294967295, 4294967295, 4294967295, 4294967295, 4294967295, 4294967295, 4294967295, 4294967295, 4294967295, 4294967295, 4294967295, 4294967295, 4294967295, 4294967295, 4294967295, 4294967295, 4294967295, 4294967295, 4294967295, 4294967295, 4294967295, 4294967295, 4294967295, 4294967295, 4294967295, 4294967295, 4294967295, 4294967295, 4294967295, 4294967295, 4294967295, 4294967295, 4294967295, 4294967295, 4294967295, 4294967295, 4294967295, 4294967295, 4294967295, 4294967295, 4294967295, 4294967295, 4294967295, 4294967295, 4294967295, 4294967295, 4294967295, 4294967295, 4294967295, 4294967295, 0, 0, 0, 0, 4294967295, 4294967295, 4294967295, 4294967295, 4294967295, 4294967295, 4294967295, 4294967295, 4294967295, 4294967295, 4294967295, 4294967295, 4294967295, 4294967295, 4294967295, 4294967295, 4294967295, 4294967295, 4294967295, 4294967295, 4294967295, 4294967295, 4294967295, 4294967295, 4294967295, 4294967295, 4294967295, 4294967295, 4294967295, 4294967295, 4294967295, 4294967295, 4294967295, 4294967295, 4294967295, 4294967295, 4294967295, 4294967295, 4294967295, 4294967295, 4294967295, 4294967295, 4294967295, 4294967295, 4294967295, 4294967295, 4294967295, 4294967295, 4294967295, 4294967295, 0, 0, 0, 0, 4294967295, 4294967295, 4294967295, 4294967295, 4294967295, 4294967295, 4294967295, 4294967295, 4294967295, 4294967295, 4294967295, 4294967295, 4294967295, 4294967295, 4294967295, 4294967295, 4294967295, 4294967295, 4294967295, 4294967295, 4294967295, 4294967295, 4294967295, 4294967295, 4294967295, 4294967295, 4294967295, 4294967295, 4294967295, 4294967295, 4294967295, 4294967295, 4294967295, 4294967295, 4294967295, 4294967295, 4294967295, 4294967295, 4294967295, 4294967295, 4294967295, 4294967295, 4294967295, 4294967295, 4294967295, 4294967295, 4294967295, 4294967295, 4294967295, 4294967295, 0, 0, 0, 0, 4294967295, 4294967295, 4294967295, 4294967295, 4294967295, 4294967295, 4294967295, 4294967295, 4294967295, 4294967295, 4294967295, 4294967295, 4294967295, 4294967295, 4294967295, 4294967295, 4294967295, 4294967295, 4294967295, 4294967295, 4294967295, 4294967295, 4294967295, 4294967295, 4294967295, 4294967295, 4294967295, 4294967295, 4294967295, 4294967295, 4294967295, 4294967295, 4294967295, 4294967295, 4294967295, 4294967295, 4294967295, 4294967295, 4294967295, 4294967295, 4294967295, 4294967295, 4294967295, 4294967295, 4294967295, 4294967295, 4294967295, 4294967295, 4294967295, 4294967295, 0, 0, 0, 0, 4294967295, 4294967295, 4294967295, 4294967295, 4294967295, 4294967295, 4294967295, 4294967295, 4294967295, 4294967295, 4294967295, 4294967295, 4294967295, 4294967295, 4294967295, 4294967295, 4294967295, 4294967295, 4294967295, 4294967295, 4294967295, 4294967295, 4294967295, 4294967295, 4294967295, 4294967295, 4294967295, 4294967295, 4294967295, 4294967295, 4294967295, 4294967295, 4294967295, 4294967295, 4294967295, 4294967295, 4294967295, 4294967295, 4294967295, 4294967295, 4294967295, 4294967295, 4294967295, 4294967295, 4294967295, 4294967295, 4294967295, 4294967295, 4294967295, 4294967295, 0, 0, 0, 0, 4294967295, 4294967295, 4294967295, 4294967295, 4294967295, 4294967295, 4294967295, 4294967295, 4294967295, 4294967295, 4294967295, 4294967295, 4294967295, 4294967295, 4294967295, 4294967295, 4294967295, 4294967295, 4294967295, 4294967295, 4294967295, 4294967295, 4294967295, 4294967295, 4294967295, 4294967295, 4294967295, 4294967295, 4294967295, 4294967295, 4294967295, 4294967295, 4294967295, 4294967295, 4294967295, 4294967295, 4294967295, 4294967295, 4294967295, 4294967295, 4294967295, 4294967295, 4294967295, 4294967295, 4294967295, 4294967295, 4294967295, 4294967295, 4294967295, 4294967295, 0, 0, 0, 0], 19 "custom trig out":u32[](graph)=[4294967295, 4294967295, 4294967295, 4294967295, 4294967295, 4294967295, 4294967295, 4294967295, 4294967295, 4294967295, 4294967295, 4294967295, 4294967295, 4294967295, 4294967295, 4294967295, 4294967295, 4294967295, 4294967295, 4294967295, 4294967295, 4294967295, 4294967295, 4294967295, 4294967295, 4294967295, 4294967295, 4294967295, 4294967295, 4294967295, 4294967295, 4294967295, 4294967295, 4294967295, 4294967295, 4294967295, 4294967295, 4294967295, 4294967295, 4294967295, 4294967295, 4294967295, 4294967295, 4294967295, 4294967295, 4294967295, 4294967295, 4294967295, 4294967295, 4294967295, 4294967295, 4294967295, 4294967295, 4294967295, 0, 0, 0, 0, 0, 0, 0, 0, 0, 0, 0, 0, 0, 0, 0, 0, 0, 0, 0, 0, 0, 0, 0, 0, 0, 0, 0, 0, 0, 0, 0, 0, 0, 0, 0, 0, 0, 0, 0, 0, 0, 0, 0, 0, 0, 0, 0, 0, 0, 0, 0, 0, 0, 0, 4294967295, 4294967295, 4294967295, 4294967295, 4294967295, 4294967295, 4294967295, 4294967295, 4294967295, 4294967295, 4294967295, 4294967295, 4294967295, 4294967295, 4294967295, 4294967295, 4294967295, 4294967295, 4294967295, 4294967295, 4294967295, 4294967295, 4294967295, 4294967295, 4294967295, 4294967295, 4294967295, 4294967295, 4294967295, 4294967295, 4294967295, 4294967295, 4294967295, 4294967295, 4294967295, 4294967295, 4294967295, 4294967295, 4294967295, 4294967295, 4294967295, 4294967295, 4294967295, 4294967295, 4294967295, 4294967295, 4294967295, 4294967295, 4294967295, 4294967295, 4294967295, 4294967295, 4294967295, 4294967295, 0, 0, 0, 0, 0, 0, 0, 0, 0, 0, 0, 0, 0, 0, 0, 0, 0, 0, 0, 0, 0, 0, 0, 0, 0, 0, 0, 0, 0, 0, 0, 0, 0, 0, 0, 0, 0, 0, 0, 0, 0, 0, 0, 0, 0, 0, 0, 0, 0, 0, 0, 0, 0, 0, 4294967295, 4294967295, 4294967295, 4294967295, 4294967295, 4294967295, 4294967295, 4294967295, 4294967295, 4294967295, 4294967295, 4294967295, 4294967295, 4294967295, 4294967295, 4294967295, 4294967295, 4294967295, 4294967295, 4294967295, 4294967295, 4294967295, 4294967295, 4294967295, 4294967295, 4294967295, 4294967295, 4294967295, 4294967295, 4294967295, 4294967295, 4294967295, 4294967295, 4294967295, 4294967295, 4294967295, 4294967295, 4294967295, 4294967295, 4294967295, 4294967295, 4294967295, 4294967295, 4294967295, 4294967295, 4294967295, 4294967295, 4294967295, 4294967295, 4294967295, 4294967295, 4294967295, 4294967295, 4294967295, 0, 0, 0, 0, 0, 0, 0, 0, 0, 0, 0, 0, 0, 0, 0, 0, 0, 0, 0, 0, 0, 0, 0, 0, 0, 0, 0, 0, 0, 0, 0, 0, 0, 0, 0, 0, 0, 0, 0, 0, 0, 0, 0, 0, 0, 0, 0, 0, 0, 0, 0, 0, 0, 0, 4294967295, 4294967295, 4294967295, 4294967295, 4294967295, 4294967295, 4294967295, 4294967295, 4294967295, 4294967295, 4294967295, 4294967295, 4294967295, 4294967295, 4294967295, 4294967295, 4294967295, 4294967295, 4294967295, 4294967295, 4294967295, 4294967295, 4294967295, 4294967295, 4294967295, 4294967295, 4294967295, 4294967295, 4294967295, 4294967295, 4294967295, 4294967295, 4294967295, 4294967295, 4294967295, 4294967295, 4294967295, 4294967295, 4294967295, 4294967295, 4294967295, 4294967295, 4294967295, 4294967295, 4294967295, 4294967295, 4294967295, 4294967295, 4294967295, 4294967295, 4294967295, 4294967295, 4294967295, 4294967295, 0, 0, 0, 0, 0, 0, 0, 0, 0, 0, 0, 0, 0, 0, 0, 0, 0, 0, 0, 0, 0, 0, 0, 0, 0, 0, 0, 0, 0, 0, 0, 0, 0, 0, 0, 0, 0, 0, 0, 0, 0, 0, 0, 0, 0, 0, 0, 0, 0, 0, 0, 0, 0, 0, 0, 0, 0, 0, 0, 0, 0, 0, 0, 0, 0, 0, 0, 0, 0, 0, 0, 0, 0, 0, 0, 0, 0, 0, 0, 0, 0, 0, 0, 0, 0, 0, 0, 0, 0, 0, 0, 0, 0, 0, 0, 0, 0, 0, 0, 0, 0, 0, 0, 0, 0, 0, 0, 0, 0, 0, 0, 0, 0, 0, 0, 0, 0, 0, 0, 0, 0, 0, 0, 0, 0, 0, 0, 0, 0, 0, 0, 0, 0, 0, 0, 0, 0, 0, 0, 0, 0, 0, 0, 0, 0, 0, 0, 0, 0, 0, 0, 0, 0, 0, 0, 0, 0, 0, 0, 0, 0, 0, 0, 0, 0, 0, 0, 0, 0, 0, 0, 0, 0, 0, 0, 0, 0, 0, 0, 0, 0, 0, 0, 0, 0, 0, 0, 0, 0, 0, 0, 0, 0, 0, 0, 0, 0, 0, 0, 0, 0, 0, 0, 0, 0, 0, 0, 0, 0, 0, 0, 0, 0, 0, 0, 0, 0, 0, 0, 0, 0, 0, 0, 0, 0, 0, 0, 0, 0, 0, 0, 0, 0, 0, 0, 0, 0, 0, 0, 0, 0, 0, 0, 0, 0, 0, 0, 0, 0, 0, 0, 0, 0, 0, 0, 0, 0, 0, 0, 0, 0, 0, 0, 0, 0, 0, 0, 0, 0, 0, 0, 0, 0, 0, 0, 0, 0, 0, 0, 0, 0, 0, 0, 0, 0, 0, 0, 0, 0, 0, 0, 0, 0, 0, 0, 0, 0, 0, 0, 0, 0, 0, 0, 0, 0, 0, 0, 0, 0, 0, 0, 0, 0, 0, 0, 0, 0, 0, 0, 0, 0, 0, 0, 0, 0, 0, 0, 0, 0, 0, 0, 0, 0, 0, 0, 0, 0, 0, 0, 0, 0, 0, 0, 0, 0, 0, 0, 0, 0, 0, 0, 0, 0, 0, 0, 0, 0, 0, 0, 0, 0, 0, 0, 0, 0, 0, 0, 0, 0, 0, 0, 0, 0, 0, 0, 0, 0, 0, 0, 0, 0, 0, 0, 0, 0, 0, 0, 0, 0, 0, 0, 0, 0, 0, 0, 0, 0, 0, 0, 0, 0, 0, 0, 0, 0, 0, 0, 0, 0, 0, 0, 0, 0, 0, 0, 0, 0, 0, 0, 0, 0, 0, 0, 0, 0, 0, 0, 0, 0, 0, 0, 0, 0, 0, 0, 0, 0, 0, 0, 0, 0, 0, 0, 0, 0, 0, 0, 0, 0, 0, 0, 0, 0, 0, 0, 0, 0, 0, 0, 0, 0, 0, 0, 0, 0, 0, 0, 0, 0, 0, 0, 0, 0, 0, 0, 0, 0, 0, 0, 0, 0, 0, 0, 0, 0, 0, 0, 0, 0, 0, 0, 0, 0, 0, 0, 0, 0, 0, 0, 0, 0, 0, 0, 0, 0, 0, 0, 0, 0, 0, 0, 0, 0, 0, 0, 0, 0, 0, 0, 0, 0, 0, 0, 0, 0, 0, 0, 0, 0, 0, 0, 0, 0, 0, 0, 0, 0, 0, 0, 0, 0, 0, 0, 0, 0, 0, 0, 0, 0, 0, 0, 0, 0, 0, 0, 0, 0, 0, 0, 0, 0, 0, 0, 0, 0, 0, 0, 0, 0, 0, 0, 0, 0, 0, 0, 0, 0, 0, 0, 0, 0, 0, 0, 0, 0, 0, 0, 0, 0, 0, 0, 0, 0, 0, 0, 0, 0, 0, 0, 0, 0, 0, 0, 0, 0, 0, 0, 0, 0, 0, 0, 0, 0, 0, 0, 0, 0, 0, 0, 0, 0, 0, 0, 0, 0, 0, 0, 0, 0, 0, 0, 0, 0, 0, 0, 0, 0, 0, 0, 0, 0, 0, 0, 0, 0, 0, 0, 0, 0, 0, 0, 0, 0, 0, 0, 0, 0, 0, 0, 0, 0, 0, 0, 0, 0, 0, 0, 0, 0, 0, 0, 0, 0, 0, 0, 0, 0, 0, 0, 0, 0, 0, 0, 0, 0, 0, 0, 0, 0, 0, 0, 0, 0, 0, 0, 0, 0, 0, 0, 0, 0, 0])   [LabVIEW 2021]
uses:
  <vilib>/Analysis/1siggen.llb/Ramp Pattern by Samples.vi
  <vilib>/Analysis/NI_AALBase.lvlib
panel:
  out "size(s)":i32=1080
  # "settings for all modes"
  # "mode 0 only"
  # "mode 13 only"
  # "mode 0,2, 12 only"
  # "mode 2, 12 only"
  # "mode 0, 1, 2 only(bidir / sin scan)"
  # "mode 1, 2 only(bidir / sin scan)"
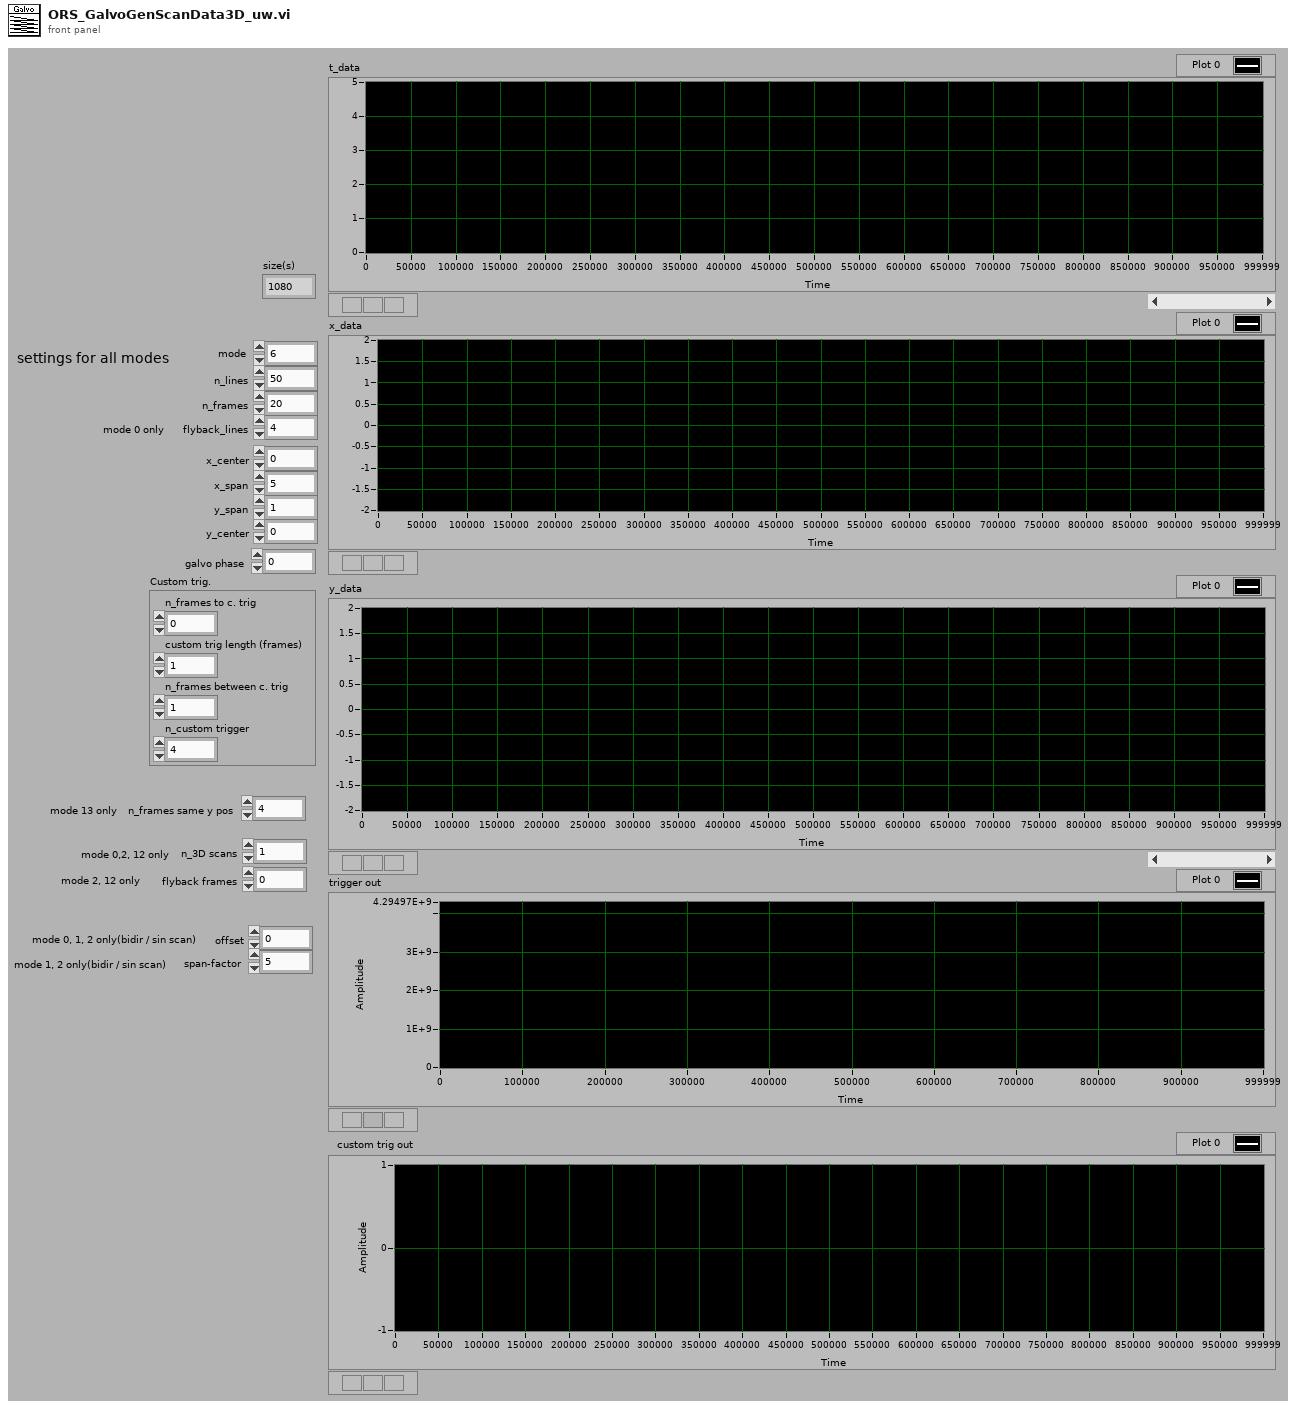
[diagram p1: front panel]
types:
  T1 = cluster{"n_frames to c. trig":i32, "custom trig length (frames)":i32, "n_frames between c. trig":i32, "n_custom trigger":i32}
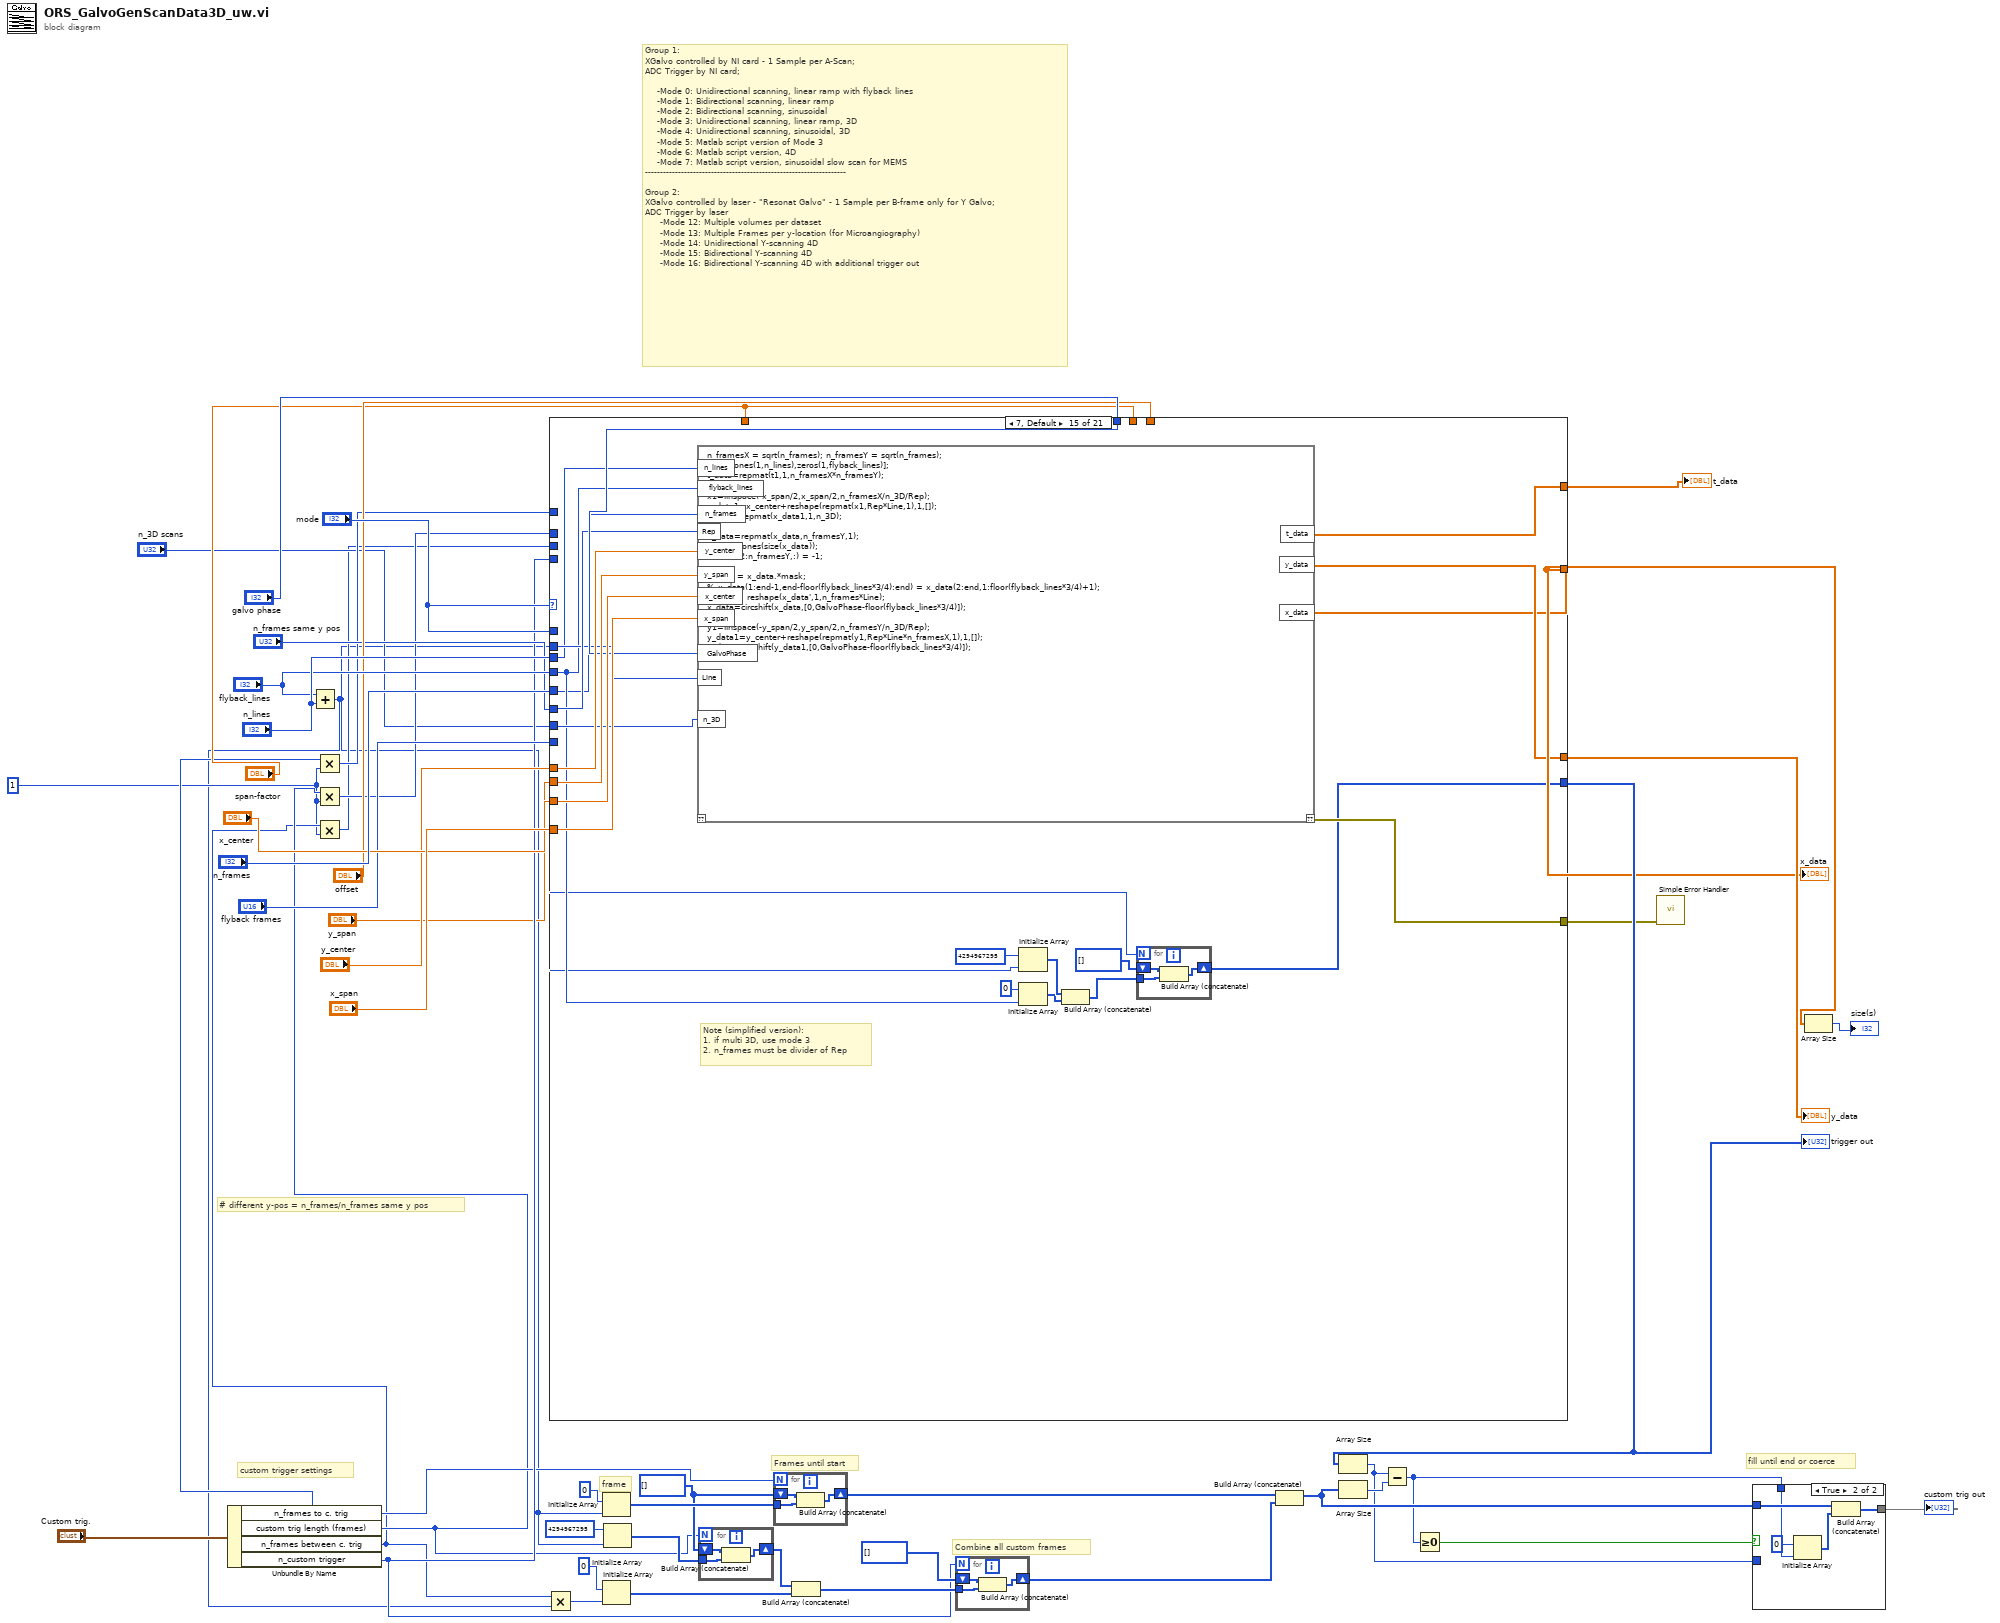
[diagram p0: block diagram]
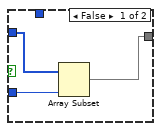
[diagram p2: hidden frame]
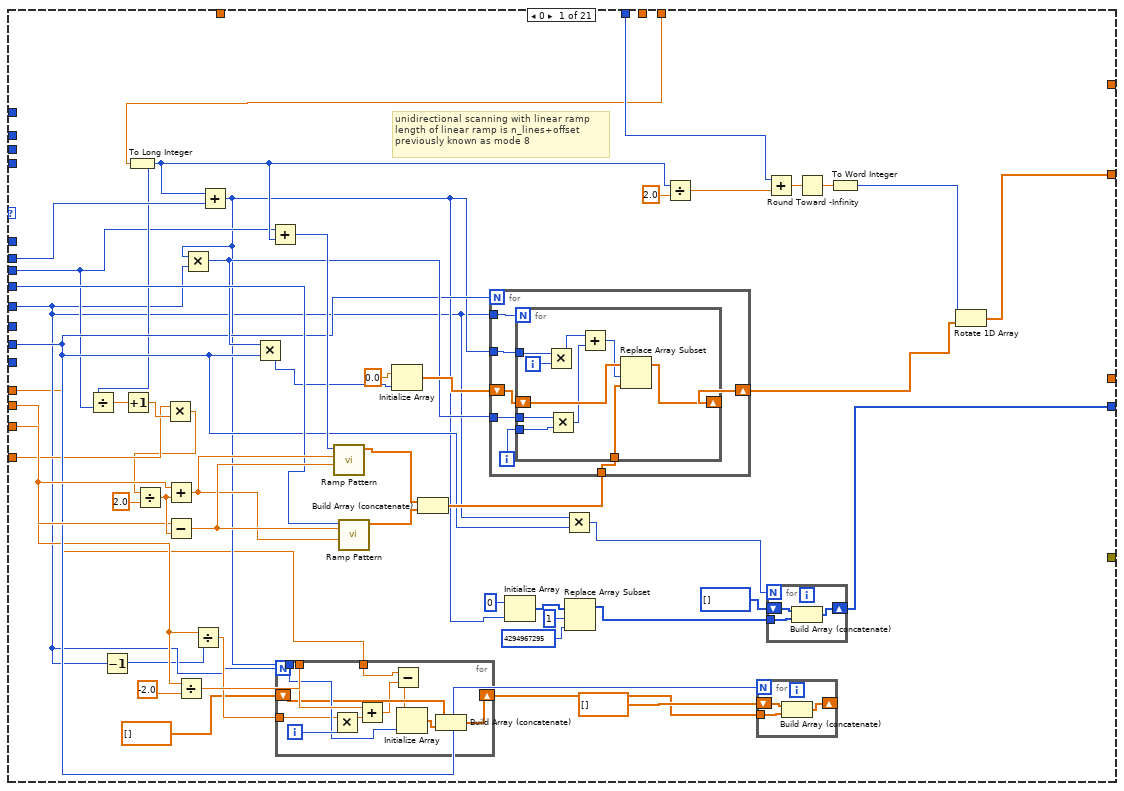
[diagram p3: hidden frame]
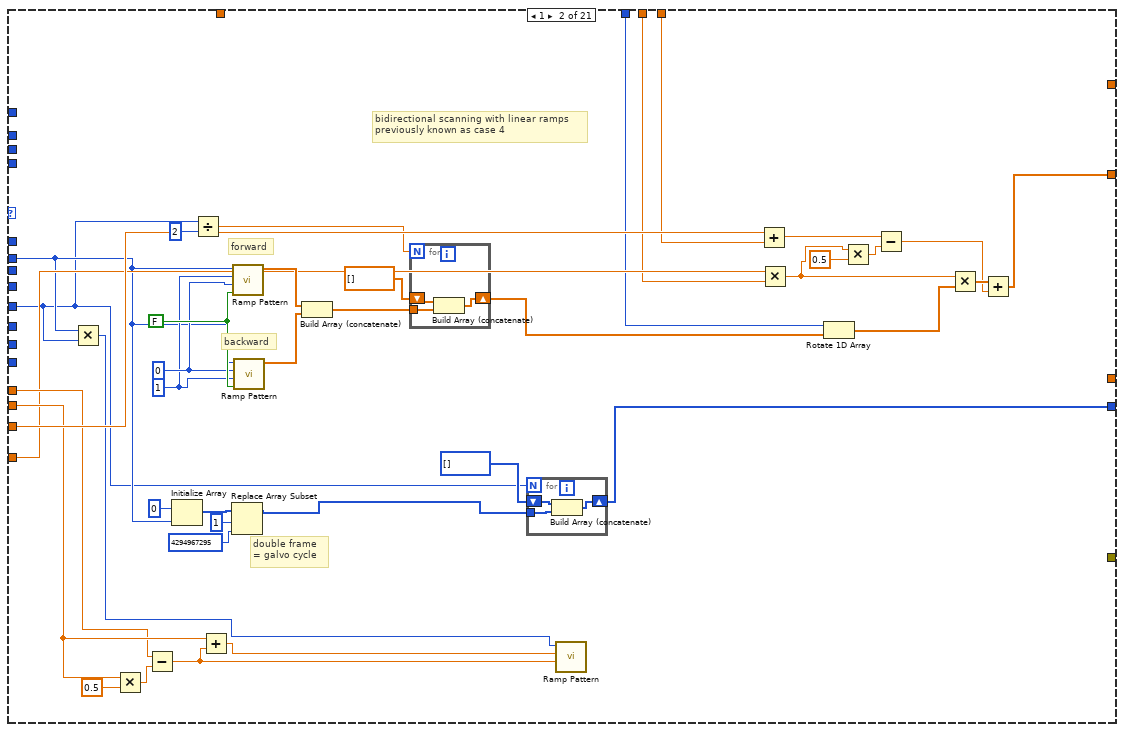
[diagram p4: hidden frame]
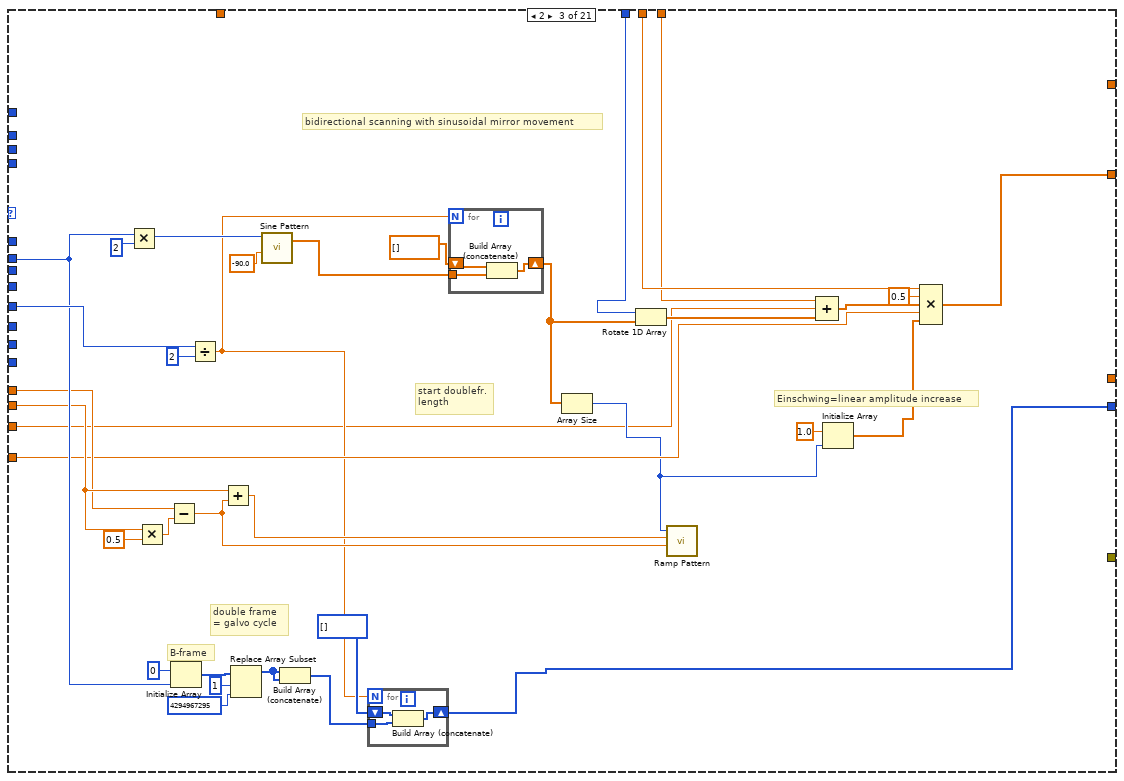
[diagram p5: hidden frame]
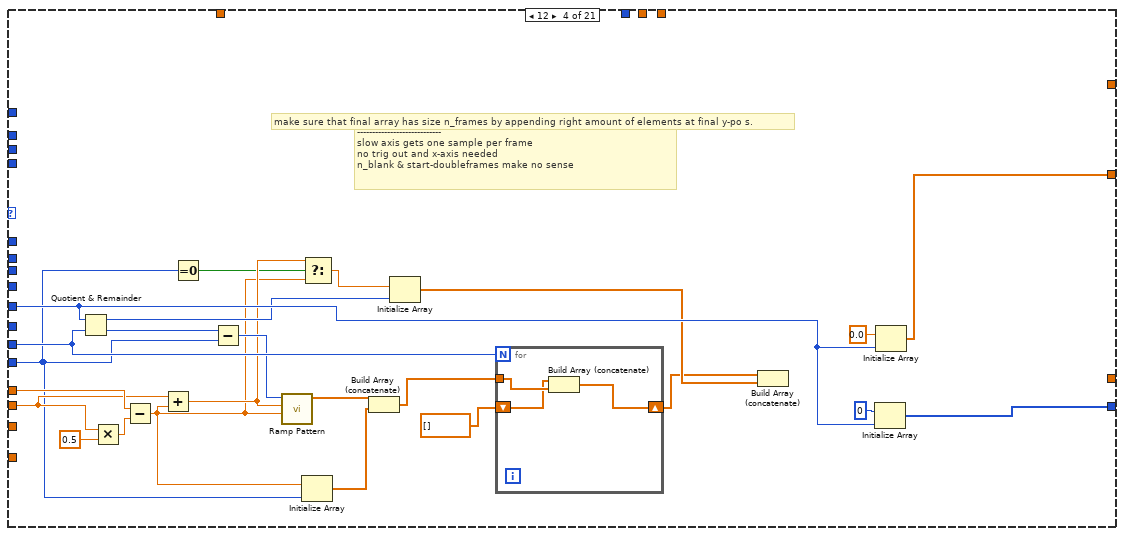
[diagram p6: hidden frame]
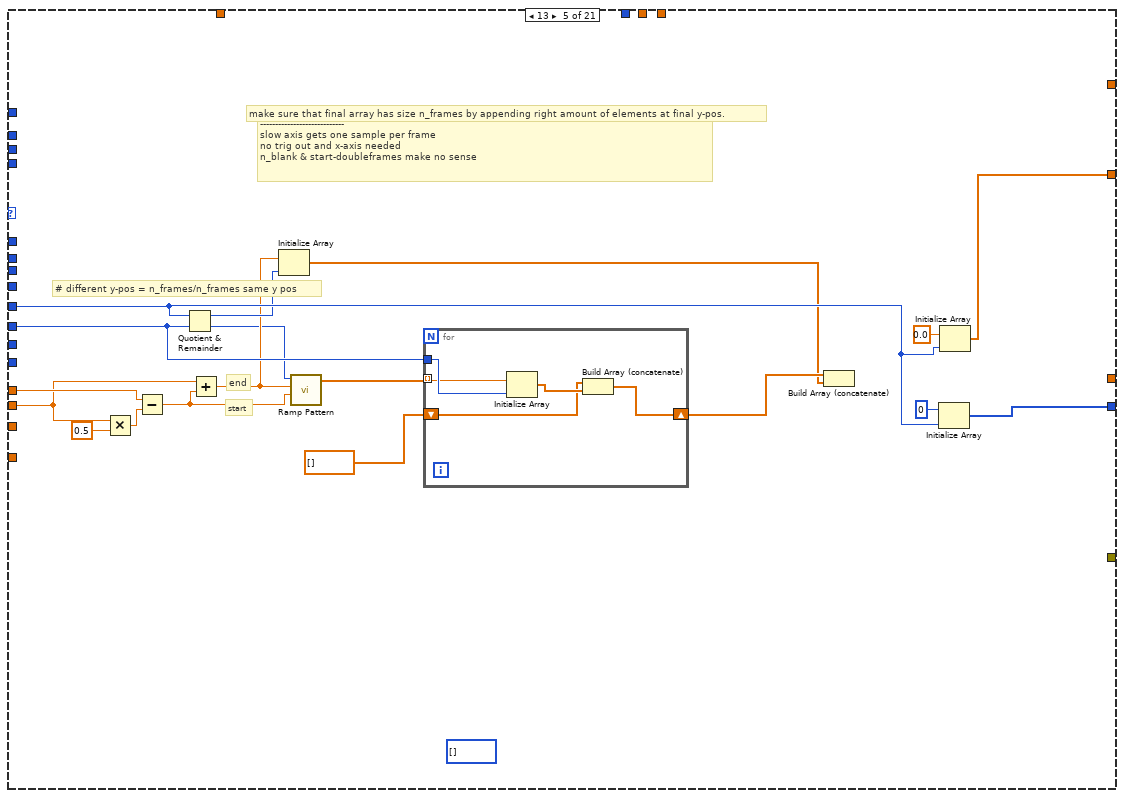
[diagram p7: hidden frame]
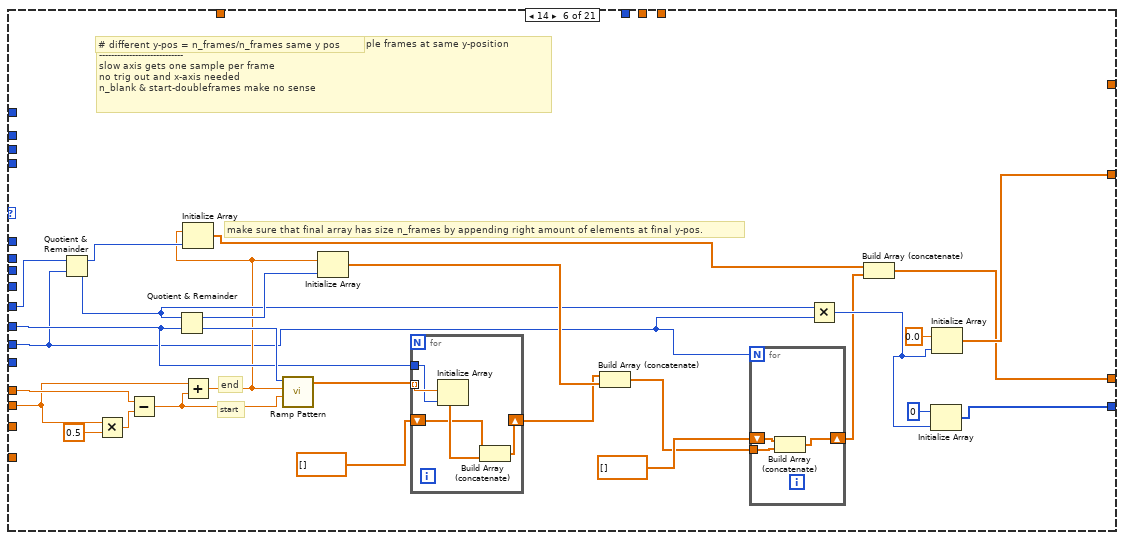
[diagram p8: hidden frame]
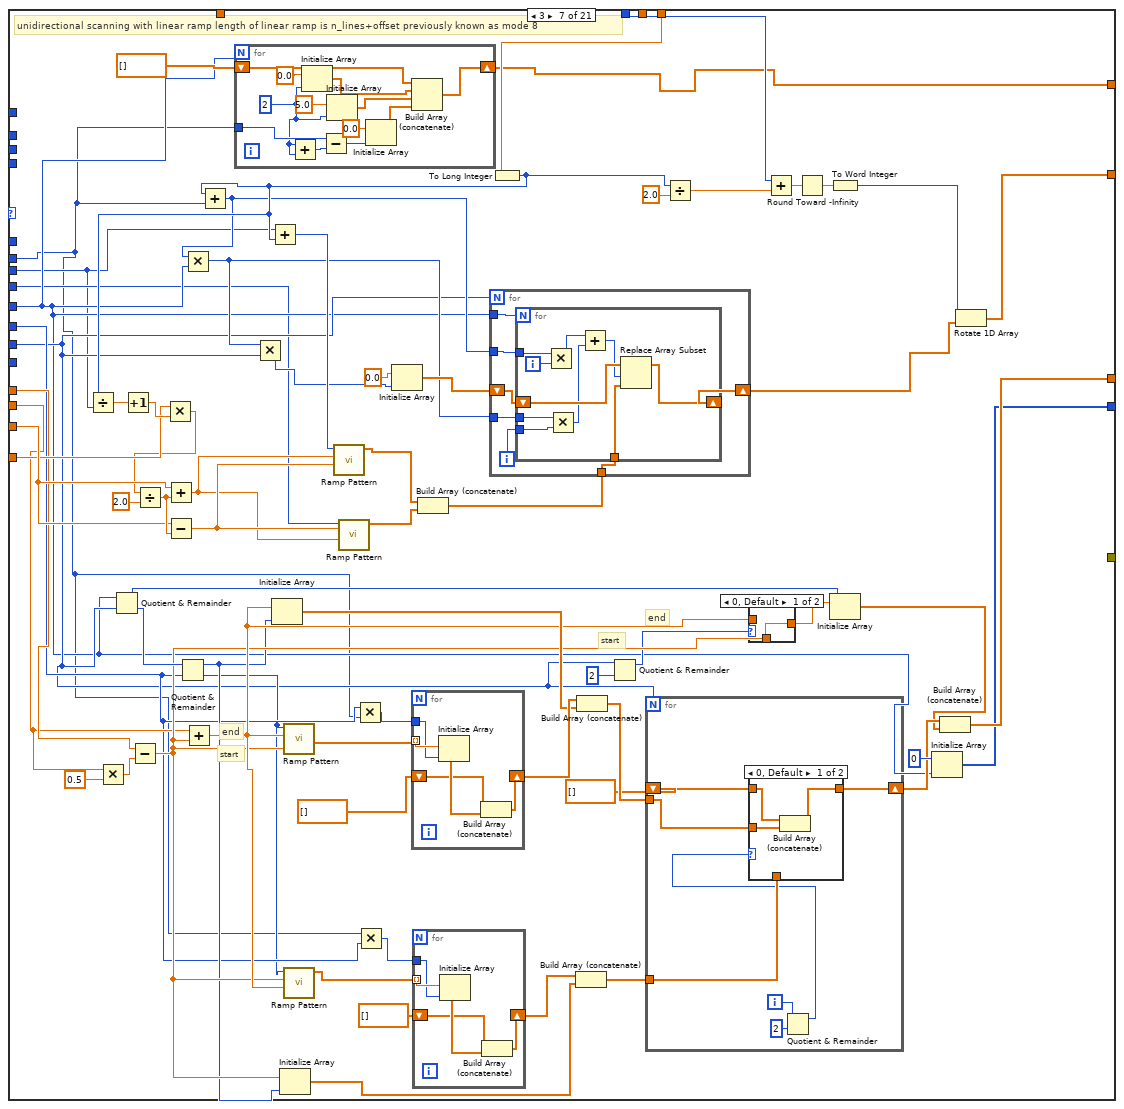
[diagram p9: hidden frame]
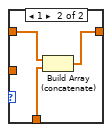
[diagram p11: hidden frame]
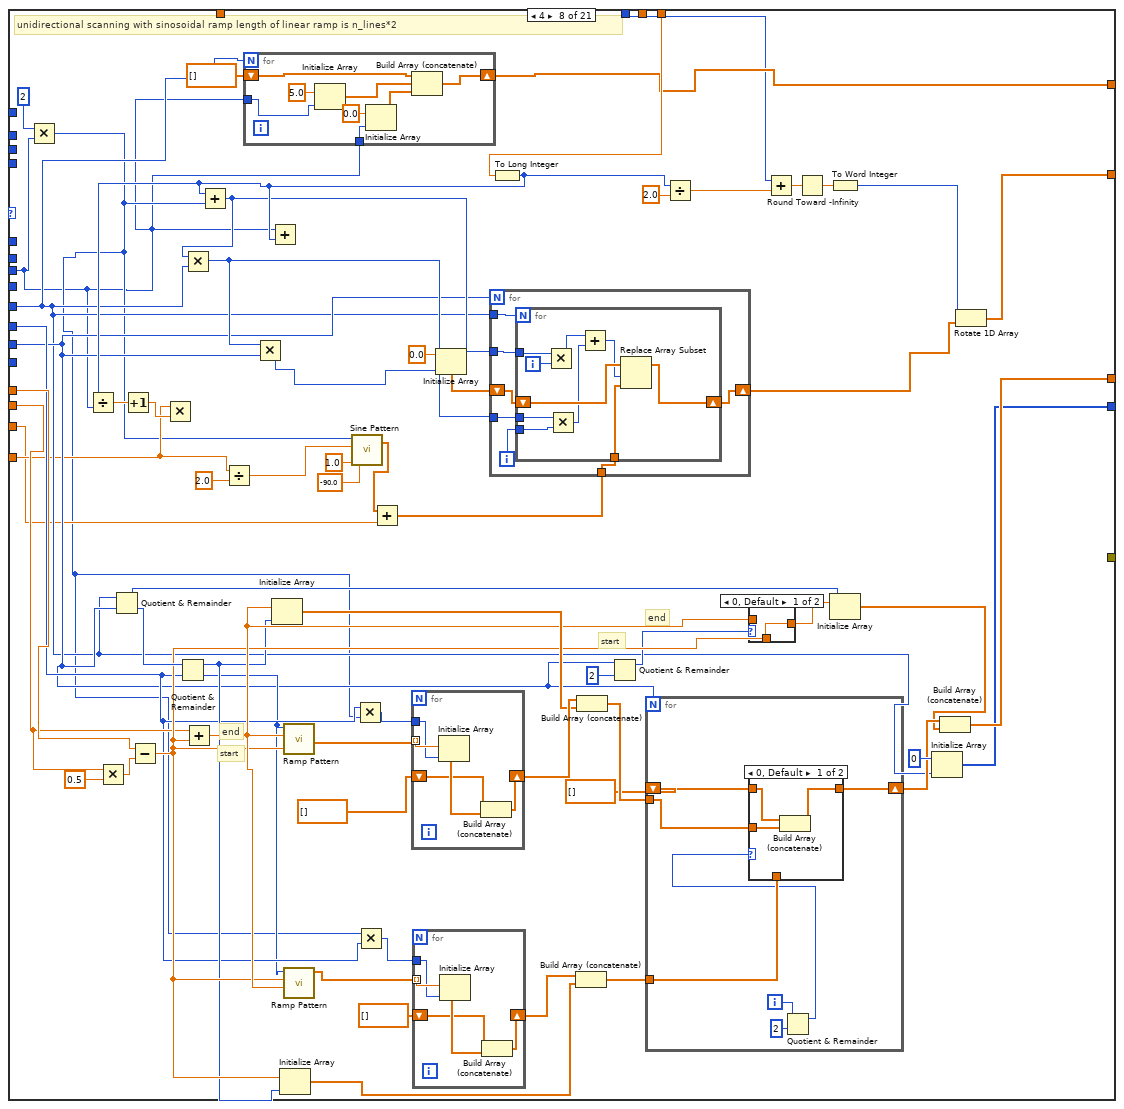
[diagram p12: hidden frame]
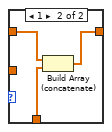
[diagram p14: hidden frame]
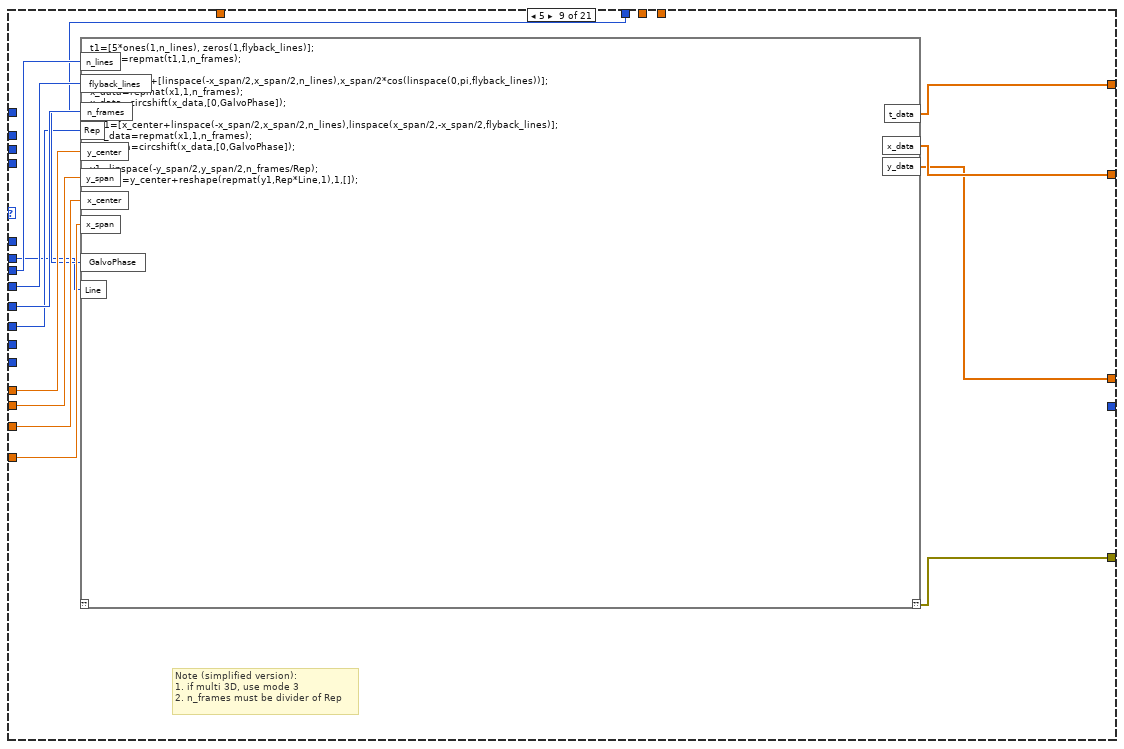
[diagram p15: hidden frame]
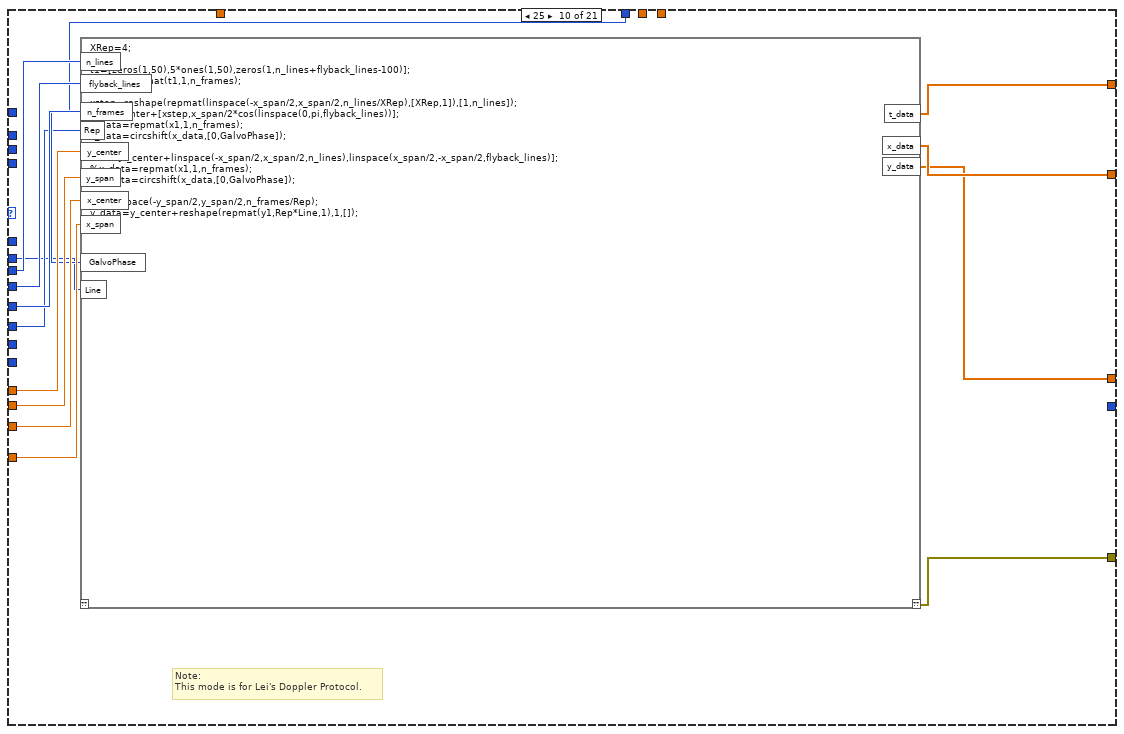
[diagram p16: hidden frame]
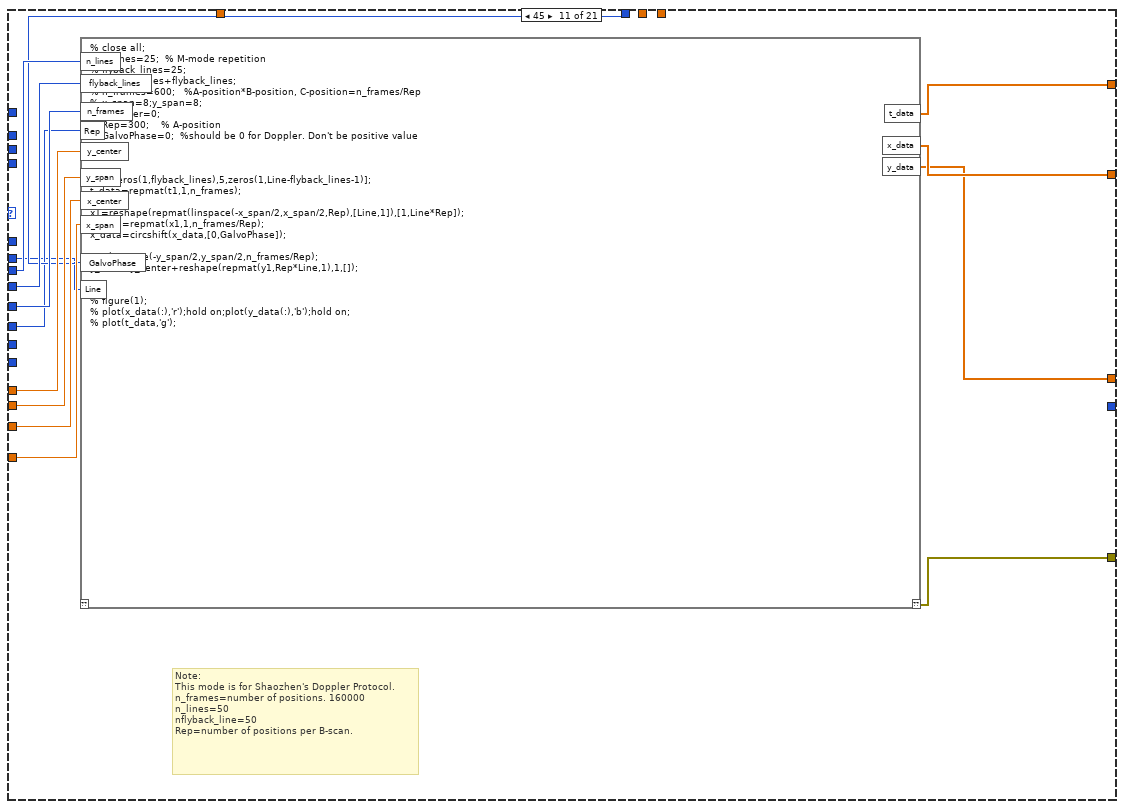
[diagram p17: hidden frame]
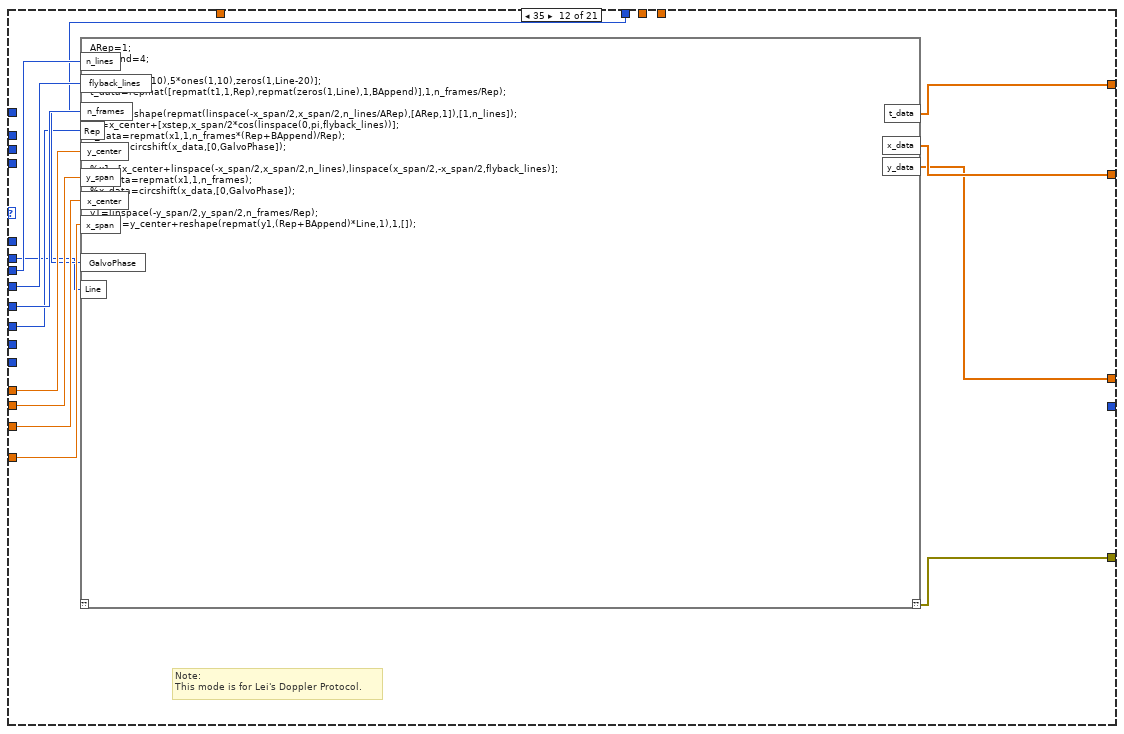
[diagram p18: hidden frame]
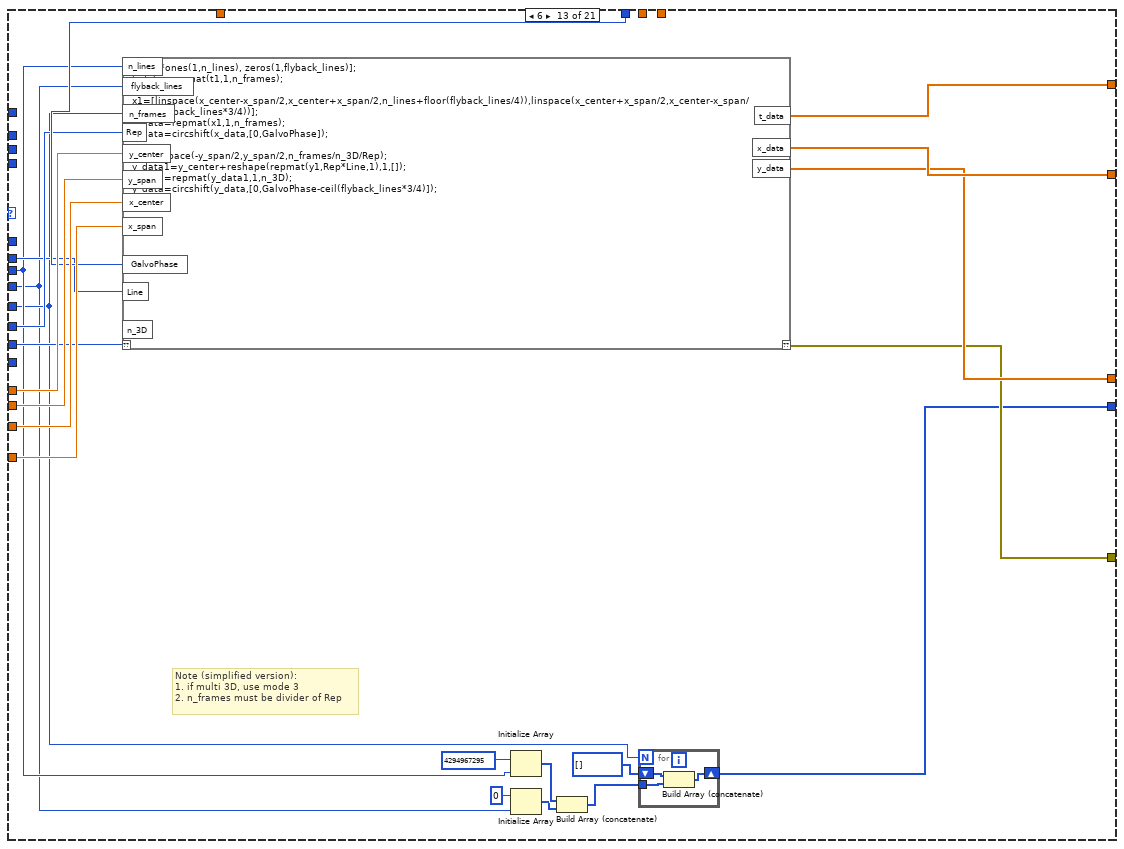
[diagram p19: hidden frame]
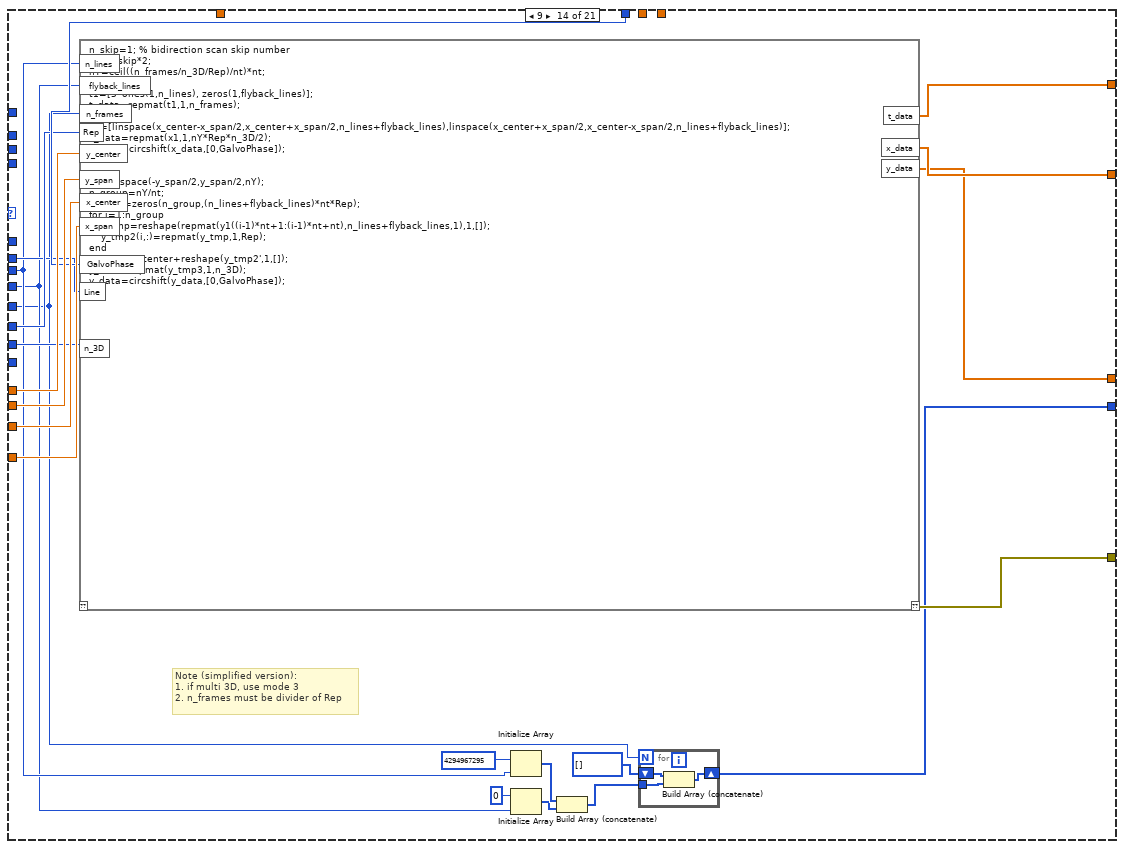
[diagram p20: hidden frame]
diagram:
  w3 = 1 ("y")
  w28 = u32[] [] ("output array")
  # "# different y-pos = n_frames/n_frames same y pos"
  # "Group 1:\nXGalvo controlled by NI card - 1 Sample per A-Scan;\nADC Trigger by NI card;\n\n    -Mode 0: Unidirectional scanning, linear ramp with flyback lines\n    -Mode 1: Bidirectional scanning, linear ramp\n    -Mode 2: Bidirectional scanning, sinusoidal\n    -Mode 3: Unidirectional scanning, linear ramp, 3D\n    -Mode 4: Unidirectional scanning, sinusoidal, 3D\n    -Mode 5: Matlab script version of Mode 3\n    -Mode 6: Matlab script version, 4D\n    -Mode 7: Matlab script version, sinusoidal slow scan for MEMS\n-------------------------------------------------------------------\n\nGroup 2:\nXGalvo controlled by laser - \"Resonat Galvo\" - 1 Sample per B-frame only for Y Galvo;\nADC Trigger by laser\n     -Mode 12: Multiple volumes per dataset\n     -Mode 13: Multiple Frames per y-location (for Microangiography)\n     -Mode 14: Unidirectional Y-scanning 4D\n     -Mode 15: Bidirectional Y-scanning 4D\n     -Mode 16: Bidirectional Y-scanning 4D with additional trigger out"
  # "fill until end or coerce"
  # "frame"
  # "Combine all custom frames"
  # "Frames until start"
  # "custom trigger settings"
  n1 = Unbundle By Name("Custom trig.") -> ("n_frames to c. trig"=w12:i32, "custom trig length (frames)"=w10:i32, "n_frames between c. trig"=w8:i32, "n_custom trigger"=w13:i32)
  n2 = Add(x="flyback_lines", y="n_lines") -> (x+y=w1:i32)
  n3 = Multiply(x=w12, y=w3) -> (x*y=w11:i32)
  n4 = Multiply(x=w10, y=w3) -> (x*y=w9:i32)
  n5 = Multiply(x=w8, y=w3) -> (x*y=w2:i32)
  n6 = Multiply(x=w8, y=w1) -> (x*y=w37:i32)
  n7 = case shown="7, Default" "mode" {
    tunnel: "y_center" -> [w54 w157 w194 w242 w263 w282 w319 w449 w551 w565 w579 w593 w618 w643 w668 w683 w703 w723 w743 w771 w841]
    tunnel: "y_span" -> [w62 w158 w195 w241 w262 w281 w318 w448 w550 w564 w578 w592 w617 w642 w667 w682 w702 w722 w742 w770 w840]
    tunnel: [_ _ _ _ _ w272 w321 w451 w544 w558 w572 w586 w611 w636 w663 w678 w698 w718 w738 w757 w829] -> w20
    tunnel: "n_frames" -> [w56 w136 w207 w236 w252 w279 w310 w441 w553 w567 w581 w595 w598 w622 w648 w685 w705 w725 w745 w759 w812]
    tunnel: "n_lines" -> [w63 _ _ _ _ _ w307 w427 w554 w568 w582 w596 w600 w625 w649 w686 w706 w726 w746 _ _]
    tunnel: "flyback_lines" -> [w80 _ _ _ _ _ w309 _ w552 w566 w580 w594 w597 w624 w650 w684 w704 w724 w744 _ _]
    tunnel: w1 -> [w85 w139 w200 _ _ _ w306 _ w542 w556 w570 w584 w609 w634 w661 w676 w696 w716 w736 _ _]
    tunnel: [w50 w135 w180 w240 w260 w283 w320 w450 _ _ _ _ w599 w623 w647 _ w687 w707 w727 w769 w839] -> w41
    tunnel: [w51 w152 w202 w239 w259 w280 w347 w476 w545 w559 w573 w587 w612 w637 w659 w673 w694 w714 w734 w768 w811] -> w17
    tunnel: "x_center" -> [w95 w159 w179 _ _ _ w369 w431 w549 w563 w577 w591 w616 w641 w666 w681 w701 w721 w741 _ _]
    tunnel: "x_span" -> [w66 w147 w190 _ _ _ w353 w435 w548 w562 w576 w590 w615 w640 w665 w680 w700 w720 w740 _ _]
    tunnel: "mode" -> [_ _ _ _ _ _ _ _ _ _ _ _ _ _ _ _ _ _ _ _ _]
    tunnel: "span-factor" -> [_ w142 w187 _ _ _ _ _ _ _ _ _ _ _ _ _ _ _ _ _ _]
    tunnel: "offset" -> [w53 w143 w186 _ _ _ w349 w478 _ _ _ _ _ _ _ _ _ _ _ _ _]
    tunnel: "galvo phase" -> [w77 w144 w185 _ _ _ w346 w437 w547 w561 w575 w589 w614 w639 w664 w679 w699 w719 w739 _ _]
    tunnel: "span-factor" -> [_ _ _ _ _ _ _ _ _ _ _ _ _ _ _ _ _ _ _ _ _]
    tunnel: "n_frames same y pos" -> [_ _ _ _ w255 w277 w315 w446 w543 w557 w571 w585 w610 w635 w662 w677 w697 w717 w737 w766 w837]
    tunnel: "n_3D scans" -> [w70 _ _ w231 _ w271 w312 w443 _ _ _ _ w608 w633 w657 w675 w695 w715 w735 w747 w820]
    tunnel: "flyback frames" -> [_ _ _ w222 _ _ _ _ _ _ _ _ _ _ _ _ _ _ _ _ _]
    tunnel: w11 -> [_ _ _ _ _ _ _ _ _ _ _ _ _ _ _ _ _ _ _ _ w819]
    tunnel: w9 -> [_ _ _ _ _ _ _ _ _ _ _ _ _ _ _ _ _ _ _ _ w817]
    tunnel: w2 -> [_ _ _ _ _ _ _ _ _ _ _ _ _ _ _ _ _ _ _ _ w816]
    tunnel: w13 -> [_ _ _ _ _ _ _ _ _ _ _ _ _ _ _ _ _ _ _ _ w818]
    tunnel: [_ _ _ _ _ _ w308 w440 w546 w560 w574 w588 w613 w638 w660 w674 w692 w708 w728 _ _] -> w7
    tunnel: [_ _ _ _ _ _ _ _ w541 w555 w569 w583 w607 w632 w658 w672 w693 w713 w733 _ _] -> w5
    frame 0 {
      # "unidirectional scanning with linear ramp\nlength of linear ramp is n_lines+offset \npreviously known as mode 8"
      n8 = Decrement(x=w56) -> (x-1=w55:i32)
      n9 = To Long Integer(number=w53) -> (32bit integer=w64:i32)
      n10 = Divide(x=w64, y=w63) -> (x/y=w68:dbl)
      n11 = Increment(x=w68) -> (x+1=w67:dbl)
      n12 = Multiply(x=w66, y=w67) -> (x*y=w65:dbl)
      n13 = Divide(x=w65, y=2.0) -> (x/y=w97:dbl)
      n14 = Add(x=w95, y=w97) -> (x+y=w93:dbl)
      n15 = Subtract(x=w95, y=w97) -> (x-y=w94:dbl)
      n16 = Divide(x=w62, y=-2.0) -> (x/y=w61:dbl)
      n17 = Divide(x=w62, y=w55) -> (x/y=w58:dbl)
      n18 = Add(x=w64, y=w85) -> (x+y=w60:i32)
      n19 = Multiply(x=w60, y=w56) -> (x*y=w72:i32)
      n20 = Multiply(x=w72, y=w70) -> (x*y=w73:u32)
      n21 = Add(x=w63, y=w64) -> (x+y=w81:i32)
      n22 = for {
        N: w56 -> [_]
        tunnel: w61 -> [w108]
        tunnel: w60 -> [w107]
        shift-right: [w103] -> w59
        shift-left: dbl[] [] -> [w104]
        tunnel: w58 -> [w105]
        tunnel: w54 -> [w101]
        i -> [w110]
        n23 = Multiply(x=w105, y=w110) -> (x*y=w109:dbl)
        n24 = Add(x=w108, y=w109) -> (x+y=w100:dbl)
        n25 = Subtract(x=w101, y=w100) -> (x-y=w102:dbl)
        n26 = Initialize Array(w102, w107) -> (w106:dbl[])
        n27 = Build Array (concatenate)(w104, w106) -> (w103:dbl[])
      }
      n28 = call-poly <vilib>:"Ramp Pattern.vi"("start"=w94, "end"=w93, "samples"=w81) -> ("Ramp Pattern"=w84:dbl[])  [unwired: 7 in, 1 out]
      n29 = call-poly <vilib>:"Ramp Pattern.vi"("start"=w93, "end"=w94, "samples"=w80) -> ("Ramp Pattern"=w83:dbl[])  [unwired: 7 in, 1 out]
      n30 = Initialize Array(0.0 ("element"), w73) -> (w92:dbl[])
      n31 = Build Array (concatenate)(w84, w83) -> (w82:dbl[])
      n32 = for {
        N: w70 -> [_]
        tunnel: w56 -> [w118]
        tunnel: w60 -> [w117]
        tunnel: w82 -> [w116]
        shift-right: [w119] -> w52
        shift-left: w92 -> [w120]
        tunnel: w72 -> [w114]
        i -> [w115]
        n33 = for {
          N: w118 -> [_]
          tunnel: w117 -> [w130]
          shift-right: [w127] -> w119
          shift-left: w120 -> [w128]
          tunnel: w116 -> [w126]
          tunnel: w115 -> [w125]
          tunnel: w114 -> [w124]
          i -> [w129]
          n34 = Multiply(x=w130, y=w129) -> (x*y=w122:i32)
          n35 = Multiply(x=w124, y=w125) -> (x*y=w123:i32)
          n36 = Add(x=w122, y=w123) -> (x+y=w121:i32)
          n37 = Replace Array Subset(array=w128, new element=w126, index=w121) -> (w127:dbl[])
        }
      }
      n38 = Initialize Array(u32 0 ("foo"), w60) -> (w88:u32[])
      n39 = Multiply(x=w56, y=w70) -> (x*y=w71:u32)
      n40 = Replace Array Subset(array=w88, new element=u32 4294967295 ("new element/subarray"), index=1) -> (w87:u32[])
      n41 = Divide(x=w64, y=2.0) -> (x/y=w78:dbl)
      n42 = for {
        N: w70 -> [_]
        shift-right: [w112] -> _
        shift-left: dbl[] [] -> [w113]
        tunnel: w59 -> [w111]
        n43 = Build Array (concatenate)(w113, w111) -> (w112:dbl[])
      }
      n44 = Add(x=w77, y=w78) -> (x+y=w76:dbl)
      n45 = for {
        N: w71 -> [_]
        shift-right: [w132] -> w50
        shift-left: u32[] [] ("output array") -> [w133]
        tunnel: w87 -> [w131]
        n46 = Build Array (concatenate)(w133, w131) -> (w132:u32[])
      }
      n47 = Round Toward -Infinity(1:w76) -> (0:w75:dbl)
      n48 = To Word Integer(number=w75) -> (16bit integer=w74:i16)
      n49 = Rotate 1D Array(1:w52, 2:w74) -> (0:w51:dbl[])
    }
    frame 1 {
      w170 = 1
      w171 = 0
      w172 = FALSE ("exclude end?")
      # "double frame \n= galvo cycle"
      # "backward"
      # "forward"
      # "bidirectional scanning with linear ramps\npreviously known as case 4"
      n50 = Multiply(x=w139, y=w136) -> (x*y=w138:i32)
      n51 = Multiply(x=w158, y=0.5) -> (x*y=w162:dbl)
      n52 = Subtract(x=w157, y=w162) -> (x-y=w154:dbl)
      n53 = Initialize Array(u32 0 ("foo"), w139) -> (w156:u32[])
      n54 = Divide(x=w136, y=2) -> (x/y=w141:dbl)
      n55 = Add(x=w158, y=w154) -> (x+y=w160:dbl)
      n56 = Replace Array Subset(array=w156, new element=u32 4294967295 ("new element/subarray"), index=1) -> (w134:u32[])
      n57 = call-poly <vilib>:"Ramp Pattern.vi"("exclude end?"=w172, "start"=w171, "end"=w170, "samples"=w139) -> ("Ramp Pattern"=w169:dbl[])  [unwired: 6 in, 1 out]
      n58 = call-poly <vilib>:"Ramp Pattern.vi"("exclude end?"=w172, "start"=w170, "end"=w171, "samples"=w139) -> ("Ramp Pattern"=w168:dbl[])  [unwired: 6 in, 1 out]
      n59 = Build Array (concatenate)(w169, w168) -> (w155:dbl[])
      n60 = for {
        N: w141 -> [_]
        shift-right: [w177] -> w145
        shift-left: dbl[] [] ("appended array") -> [w178]
        tunnel: w155 -> [w176]
        n61 = Build Array (concatenate)(w178, w176) -> (w177:dbl[])
      }
      n62 = for {
        N: w136 -> [_]
        shift-right: [w174] -> w135
        shift-left: u32[] [] ("output array") -> [w175]
        tunnel: w134 -> [w173]
        n63 = Build Array (concatenate)(w175, w173) -> (w174:u32[])
      }
      n64 = call-poly <vilib>:"Ramp Pattern.vi"("start"=w154, "end"=w160, "samples"=w138) -> ()  [unwired: 7 in, 2 out]
      n65 = Add(x=w159, y=w143) -> (x+y=w151:dbl)
      n66 = Multiply(x=w147, y=w142) -> (x*y=w146:dbl)
      n67 = Rotate 1D Array(1:w145, 2:w144) -> (0:w140:dbl[])
      n68 = Multiply(x=w146, y=0.5) -> (x*y=w149:dbl)
      n69 = Subtract(x=w151, y=w149) -> (x-y=w150:dbl)
      n70 = Multiply(x=w146, y=w140) -> (x*y=w153:dbl[])
      n71 = Add(x=w153, y=w150) -> (x+y=w152:dbl[])
    }
    frame 2 {
      # "start doublefr.\nlength"
      # "B-frame"
      # "double frame \n= galvo cycle"
      # "Einschwing=linear amplitude increase"
      # "bidirectional scanning with sinusoidal mirror movement"
      n72 = Multiply(x=w200, y=2) -> (x*y=w184:i32)
      n73 = Multiply(x=w195, y=0.5) -> (x*y=w198:dbl)
      n74 = Subtract(x=w194, y=w198) -> (x-y=w193:dbl)
      n75 = Initialize Array(u32 0 ("foo"), w200) -> (w208:u32[])
      n76 = Divide(x=w207, y=2) -> (x/y=w183:dbl)
      n77 = Add(x=w195, y=w193) -> (x+y=w196:dbl)
      n78 = Replace Array Subset(array=w208, new element=u32 4294967295 ("new element/subarray"), index=1) -> (w211:u32[])
      n79 = call <vilib>:"Sine Pattern.vi"("phase(degrees)"=-90.0, "samples"=w184) -> ("Sinusoidal Pattern"=w205:dbl[])  [unwired: 2 in, 1 out]
      n80 = Build Array (concatenate)(w211, w211) -> (w209:u32[])
      n81 = for {
        N: w183 -> [_]
        shift-right: [w219] -> w180
        shift-left: u32[] [] ("output array") -> [w220]
        tunnel: w209 -> [w218]
        n82 = Build Array (concatenate)(w220, w218) -> (w219:u32[])
      }
      n83 = for {
        N: w183 -> [_]
        shift-right: [w216] -> w192
        shift-left: dbl[] [] -> [w217]
        tunnel: w205 -> [w215]
        n84 = Build Array (concatenate)(w217, w215) -> (w216:dbl[])
      }
      n85 = Array Size(array=w192) -> (size(s)=w181:i32)
      n86 = Rotate 1D Array(1:w192, 2:w185) -> (0:w203:dbl[])
      n87 = call-poly <vilib>:"Ramp Pattern.vi"("start"=w193, "end"=w196, "samples"=w181) -> ()  [unwired: 7 in, 2 out]
      n88 = Compound Arithmetic op=ADD(w186, w179, w203) -> (w191:dbl[])
      n89 = Initialize Array(1.0 ("element"), w181) -> (w182:dbl[])
      n90 = Compound Arithmetic op=MULTIPLY(w187, 0.5 ("value"), w191, w190, w182) -> (w202:dbl[])
    }
    frame 12 {
      # "make sure that final array has size n_frames by appending right amount of elements at final y-po s."
      # "For resonant Galvo - allows for multiple 3D scans per dataset\n----------------------------\nslow axis gets one sample per frame\nno trig out and x-axis needed\nn_blank & start-doubleframes make no sense"
      n91 = Quotient & Remainder(x=w236, y=w231) -> (x-y*floor(x/y)=w235:u32, floor(x/y)=w230:u32)
      n92 = Multiply(x=w241, y=0.5) -> (x*y=w244:dbl)
      n93 = Subtract(x=w242, y=w244) -> (x-y=w223:dbl)
      n94 = Add(x=w241, y=w223) -> (x+y=w225:dbl)
      n95 = Equal To 0?(x=w222) -> (x = 0?=w221:bool)
      n96 = Subtract(x=w230, y=w222) -> (x-y=w229:u32)
      n97 = call-poly <vilib>:"Ramp Pattern.vi"("start"=w223, "end"=w225, "samples"=w229) -> ("Ramp Pattern"=w227:dbl[])  [unwired: 7 in, 1 out]
      n98 = Initialize Array(w223, w222) -> (w228:dbl[])
      n99 = Select(t=w225, s=w221, f=w223) -> (s? t:f=w224:dbl)
      n100 = Build Array (concatenate)(w227, w228) -> (w226:dbl[])
      n101 = Initialize Array(w224, w235) -> (w234:dbl[])
      n102 = for {
        N: w231 -> [_]
        tunnel: w226 -> [w246]
        shift-right: [w247] -> w233
        shift-left: dbl[] [] -> [w245]
        n103 = Build Array (concatenate)(w245, w246) -> (w247:dbl[])
      }
      n104 = Build Array (concatenate)(w233, w234) -> ()  [unwired: 1 out]
      n105 = Initialize Array(u32 0 ("element"), w236) -> (w240:u32[])
      n106 = Initialize Array(0.0 ("element"), w236) -> (w239:dbl[])
    }
    frame 13 {
      (unwired) u32[] [] ("output array")
      # "# different y-pos = n_frames/n_frames same y pos"
      # "make sure that final array has size n_frames by appending right amount of elements at final y-pos."
      # "end"
      # "start"
      # "For resonant Galvo - Microangiography case, scan multiple frames at same y-position\n----------------------------\nslow axis gets one sample per frame\nno trig out and x-axis needed\nn_blank & start-doubleframes make no sense"
      n107 = Multiply(x=w262, y=0.5) -> (x*y=w265:dbl)
      n108 = Subtract(x=w263, y=w265) -> (x-y=w261:dbl)
      n109 = Quotient & Remainder(x=w252, y=w255) -> (x-y*floor(x/y)=w251:u32, floor(x/y)=w248:u32)
      n110 = Add(x=w262, y=w261) -> (x+y=w250:dbl)
      n111 = Initialize Array(w250, w251) -> (w249:dbl[])
      n112 = call-poly <vilib>:"Ramp Pattern.vi"("start"=w261, "end"=w250, "samples"=w248) -> ("Ramp Pattern"=w256:dbl[])  [unwired: 7 in, 1 out]
      n113 = for {
        tunnel: w256 -> [w269] mode=indexing
        tunnel: w255 -> [w270]
        shift-right: [w267] -> w253
        shift-left: dbl[] [] -> [w266]
        n114 = Initialize Array(w269, w270) -> (w268:dbl[])
        n115 = Build Array (concatenate)(w266, w268) -> (w267:dbl[])
      }
      n116 = Build Array (concatenate)(w253, w249) -> ()  [unwired: 1 out]
      n117 = Initialize Array(u32 0 ("element"), w252) -> (w260:u32[])
      n118 = Initialize Array(0.0 ("element"), w252) -> (w259:dbl[])
    }
    frame 14 {
      # "# different y-pos = n_frames/n_frames same y pos"
      # "make sure that final array has size n_frames by appending right amount of elements at final y-pos."
      # "end"
      # "start"
      # "For resonant Galvo - Microangiography case, scan multiple frames at same y-position\n----------------------------\nslow axis gets one sample per frame\nno trig out and x-axis needed\nn_blank & start-doubleframes make no sense"
      n119 = Quotient & Remainder(x=w279, y=w271) -> (x-y*floor(x/y)=w276:u32, floor(x/y)=w278:u32)
      n120 = Multiply(x=w281, y=0.5) -> (x*y=w297:dbl)
      n121 = Subtract(x=w282, y=w297) -> (x-y=w295:dbl)
      n122 = Quotient & Remainder(x=w278, y=w277) -> (x-y*floor(x/y)=w291:u32, floor(x/y)=w289:u32)
      n123 = Add(x=w281, y=w295) -> (x+y=w275:dbl)
      n124 = Initialize Array(w275, w276) -> (w274:dbl[])
      n125 = call-poly <vilib>:"Ramp Pattern.vi"("start"=w295, "end"=w275, "samples"=w289) -> ("Ramp Pattern"=w292:dbl[])  [unwired: 7 in, 1 out]
      n126 = Initialize Array(w275, w291) -> (w290:dbl[])
      n127 = for {
        tunnel: w292 -> [w305] mode=indexing
        tunnel: w277 -> [w302]
        shift-right: [w301] -> w286
        shift-left: dbl[] [] -> [w303]
        n128 = Initialize Array(w305, w302) -> (w304:dbl[])
        n129 = Build Array (concatenate)(w303, w304) -> (w301:dbl[])
      }
      n130 = Build Array (concatenate)(w286, w290) -> (w285:dbl[])
      n131 = for {
        N: w271 -> [_]
        shift-right: [w298] -> w273
        shift-left: dbl[] [] -> [w300]
        tunnel: w285 -> [w299]
        n132 = Build Array (concatenate)(w300, w299) -> (w298:dbl[])
      }
      n133 = Multiply(x=w278, y=w271) -> (x*y=w284:u32)
      n134 = Build Array (concatenate)(w274, w273) -> (w272:dbl[])
      n135 = Initialize Array(u32 0 ("element"), w284) -> (w283:u32[])
      n136 = Initialize Array(0.0 ("element"), w284) -> (w280:dbl[])
    }
    frame 3 {
      # "unidirectional scanning with linear ramp length of linear ramp is n_lines+offset previously known as mode 8"
      # "start"
      # "end"
      # "end"
      # "start"
      n137 = Multiply(x=w318, y=0.5) -> (x*y=w338:dbl)
      n138 = Quotient & Remainder(x=w310, y=w312) -> (x-y*floor(x/y)=w331:u32, floor(x/y)=w329:u32)
      n139 = Subtract(x=w319, y=w338) -> (x-y=w327:dbl)
      n140 = Quotient & Remainder(x=w329, y=w315) -> (x-y*floor(x/y)=w322:u32, floor(x/y)=w313:u32)
      n141 = Add(x=w318, y=w327) -> (x+y=w328:dbl)
      n142 = for {
        N: w310 -> [_]
        shift-right: [w383] -> w308
        shift-left: dbl[] [] -> [w380]
        tunnel: w306 -> [w377]
        w374 = 2 ("dimension size")
        n143 = Add(x=w374, y=w374) -> (x+y=w375:i32)
        n144 = Initialize Array(0.0 ("element"), w374) -> (w379:dbl[])
        n145 = Subtract(x=w377, y=w375) -> (x-y=w378:i32)
        n146 = Initialize Array(5.0 ("element"), w374) -> (w373:dbl[])
        n147 = Initialize Array(0.0 ("element"), w378) -> (w384:dbl[])
        n148 = Build Array (concatenate)(w380, w379, w373, w384) -> (w383:dbl[])
      }
      n149 = Initialize Array(w328, w322) -> (w333:dbl[])
      n150 = Initialize Array(w327, w322) -> (w332:dbl[])
      n151 = call-poly <vilib>:"Ramp Pattern.vi"("start"=w327, "end"=w328, "samples"=w313) -> ("Ramp Pattern"=w341:dbl[])  [unwired: 7 in, 1 out]
      n152 = call-poly <vilib>:"Ramp Pattern.vi"("start"=w328, "end"=w327, "samples"=w313) -> ("Ramp Pattern"=w337:dbl[])  [unwired: 7 in, 1 out]
      n153 = Multiply(x=w315, y=w306) -> (x*y=w316:u32)
      n154 = Multiply(x=w306, y=w315) -> (x*y=w314:u32)
      n155 = for {
        tunnel: w341 -> [w409] mode=indexing
        tunnel: w316 -> [w406]
        shift-right: [w405] -> w344
        shift-left: dbl[] [] -> [w407]
        n156 = Initialize Array(w409, w406) -> (w408:dbl[])
        n157 = Build Array (concatenate)(w407, w408) -> (w405:dbl[])
      }
      n158 = for {
        tunnel: w337 -> [w391] mode=indexing
        tunnel: w314 -> [w388]
        shift-right: [w387] -> w335
        shift-left: dbl[] [] -> [w389]
        n159 = Initialize Array(w391, w388) -> (w390:dbl[])
        n160 = Build Array (concatenate)(w389, w390) -> (w387:dbl[])
      }
      n161 = To Long Integer(number=w349) -> (32bit integer=w351:i32)
      n162 = Divide(x=w351, y=w307) -> (x/y=w355:dbl)
      n163 = Increment(x=w355) -> (x+1=w354:dbl)
      n164 = Multiply(x=w353, y=w354) -> (x*y=w352:dbl)
      n165 = Divide(x=w352, y=2.0) -> (x/y=w370:dbl)
      n166 = Add(x=w369, y=w370) -> (x+y=w367:dbl)
      n167 = Subtract(x=w369, y=w370) -> (x-y=w368:dbl)
      n168 = Add(x=w351, y=w306) -> (x+y=w350:i32)
      n169 = Multiply(x=w350, y=w310) -> (x*y=w356:i32)
      n170 = Multiply(x=w356, y=w312) -> (x*y=w357:u32)
      n171 = Add(x=w307, y=w351) -> (x+y=w363:i32)
      n172 = call-poly <vilib>:"Ramp Pattern.vi"("start"=w368, "end"=w367, "samples"=w363) -> ("Ramp Pattern"=w365:dbl[])  [unwired: 7 in, 1 out]
      n173 = call-poly <vilib>:"Ramp Pattern.vi"("start"=w367, "end"=w368, "samples"=w309) -> ("Ramp Pattern"=w364:dbl[])  [unwired: 7 in, 1 out]
      n174 = Initialize Array(0.0 ("element"), w357) -> (w366:dbl[])
      n175 = Build Array (concatenate)(w365, w364) -> (w317:dbl[])
      n176 = for {
        N: w312 -> [_]
        tunnel: w310 -> [w414]
        tunnel: w350 -> [w413]
        tunnel: w317 -> [w412]
        shift-right: [w415] -> w348
        shift-left: w366 -> [w416]
        tunnel: w356 -> [w410]
        i -> [w411]
        n177 = for {
          N: w414 -> [_]
          tunnel: w413 -> [w426]
          shift-right: [w423] -> w415
          shift-left: w416 -> [w424]
          tunnel: w412 -> [w422]
          tunnel: w411 -> [w421]
          tunnel: w410 -> [w420]
          i -> [w425]
          n178 = Multiply(x=w426, y=w425) -> (x*y=w418:i32)
          n179 = Multiply(x=w420, y=w421) -> (x*y=w419:i32)
          n180 = Add(x=w418, y=w419) -> (x+y=w417:i32)
          n181 = Replace Array Subset(array=w424, new element=w422, index=w417) -> (w423:dbl[])
        }
      }
      n182 = Build Array (concatenate)(w335, w332) -> (w334:dbl[])
      n183 = Build Array (concatenate)(w344, w333) -> (w345:dbl[])
      n184 = Quotient & Remainder(x=w312, y=2) -> (x-y*floor(x/y)=w325:u32)  [unwired: 1 out]
      n185 = for {
        N: w312 -> [_]
        shift-right: [w395] -> w324
        shift-left: dbl[] [] -> [w396]
        tunnel: w345 -> [w397]
        tunnel: w334 -> [w394]
        i -> [w392]
        n186 = Quotient & Remainder(x=w392, y=2) -> (x-y*floor(x/y)=w393:i32)  [unwired: 1 out]
        n187 = case shown="0, Default" w393 {
          tunnel: w397 -> [w401 _]
          tunnel: w396 -> [w400 w403]
          tunnel: [w399 w402] -> w395
          tunnel: w394 -> [_ w404]
          frame 0, Default {
            n188 = Build Array (concatenate)(w400, w401) -> (w399:dbl[])
          }
          frame 1 {
            n189 = Build Array (concatenate)(w403, w404) -> (w402:dbl[])
          }
        }
      }
      n190 = Divide(x=w351, y=2.0) -> (x/y=w361:dbl)
      n191 = case shown="0, Default" w325 {
        tunnel: w328 -> [_ w386]
        tunnel: w327 -> [w385 _]
        tunnel: [w385 w386] -> w326
        frame 0, Default {
        }
        frame 1 {
        }
      }
      n192 = Add(x=w346, y=w361) -> (x+y=w360:dbl)
      n193 = Round Toward -Infinity(1:w360) -> (0:w359:dbl)
      n194 = To Word Integer(number=w359) -> (16bit integer=w358:i16)
      n195 = Initialize Array(w326, w331) -> (w323:dbl[])
      n196 = Initialize Array(u32 0 ("element"), w310) -> (w320:u32[])
      n197 = Build Array (concatenate)(w324, w323) -> (w321:dbl[])
      n198 = Rotate 1D Array(1:w348, 2:w358) -> (0:w347:dbl[])
    }
    frame 4 {
      # "unidirectional scanning with sinosoidal ramp length of linear ramp is n_lines*2"
      # "start"
      # "end"
      # "end"
      # "start"
      n199 = Multiply(x=2 ("y"), y=w427) -> (x*y=w429:i32)
      n200 = Multiply(x=w448, y=0.5) -> (x*y=w468:dbl)
      n201 = Quotient & Remainder(x=w441, y=w443) -> (x-y*floor(x/y)=w461:u32, floor(x/y)=w459:u32)
      n202 = Subtract(x=w449, y=w468) -> (x-y=w457:dbl)
      n203 = Quotient & Remainder(x=w459, y=w446) -> (x-y*floor(x/y)=w452:u32, floor(x/y)=w444:u32)
      n204 = Add(x=w448, y=w457) -> (x+y=w458:dbl)
      n205 = Divide(x=w435, y=2.0) -> (x/y=w433:dbl)
      n206 = for {
        N: w441 -> [_]
        tunnel: w427 -> [w492]
        shift-right: [w495] -> w440
        shift-left: dbl[] [] -> [w494]
        tunnel: w427 -> [w491]
        n207 = Initialize Array(5.0 ("element"), w492) -> (w498:dbl[])
        n208 = Initialize Array(0.0 ("element"), w491) -> (w496:dbl[])
        n209 = Build Array (concatenate)(w494, w498, w496) -> (w495:dbl[])
      }
      n210 = Initialize Array(w458, w452) -> (w463:dbl[])
      n211 = Initialize Array(w457, w452) -> (w462:dbl[])
      n212 = call-poly <vilib>:"Ramp Pattern.vi"("start"=w457, "end"=w458, "samples"=w444) -> ("Ramp Pattern"=w471:dbl[])  [unwired: 7 in, 1 out]
      n213 = call-poly <vilib>:"Ramp Pattern.vi"("start"=w458, "end"=w457, "samples"=w444) -> ("Ramp Pattern"=w467:dbl[])  [unwired: 7 in, 1 out]
      n214 = call <vilib>:"Sine Pattern.vi"("cycles"=1.0, "phase(degrees)"=-90.0, "amplitude"=w433, "samples"=w429) -> ("Sinusoidal Pattern"=w432:dbl[])  [unwired: 1 out]
      n215 = Multiply(x=w446, y=w429) -> (x*y=w447:u32)
      n216 = Multiply(x=w429, y=w446) -> (x*y=w445:u32)
      n217 = Add(x=w432, y=w431) -> (x+y=w430:dbl[])
      n218 = for {
        tunnel: w471 -> [w523] mode=indexing
        tunnel: w447 -> [w520]
        shift-right: [w519] -> w474
        shift-left: dbl[] [] -> [w521]
        n219 = Initialize Array(w523, w520) -> (w522:dbl[])
        n220 = Build Array (concatenate)(w521, w522) -> (w519:dbl[])
      }
      n221 = for {
        tunnel: w467 -> [w505] mode=indexing
        tunnel: w445 -> [w502]
        shift-right: [w501] -> w465
        shift-left: dbl[] [] -> [w503]
        n222 = Initialize Array(w505, w502) -> (w504:dbl[])
        n223 = Build Array (concatenate)(w503, w504) -> (w501:dbl[])
      }
      n224 = To Long Integer(number=w478) -> (32bit integer=w480:i32)
      n225 = Divide(x=w480, y=w427) -> (x/y=w482:dbl)
      n226 = Increment(x=w482) -> (x+1=w481:dbl)
      n227 = Multiply(x=w435, y=w481) -> ()  [unwired: 1 out]
      n228 = Add(x=w480, y=w429) -> (x+y=w479:i32)
      n229 = Multiply(x=w479, y=w441) -> (x*y=w483:i32)
      n230 = Multiply(x=w483, y=w443) -> (x*y=w439:u32)
      n231 = Add(x=w427, y=w480) -> ()  [unwired: 1 out]
      n232 = Initialize Array(0.0 ("element"), w439) -> (w489:dbl[])
      n233 = for {
        N: w443 -> [_]
        tunnel: w441 -> [w528]
        tunnel: w479 -> [w527]
        tunnel: w430 -> [w526]
        shift-right: [w529] -> w477
        shift-left: w489 -> [w530]
        tunnel: w483 -> [w524]
        i -> [w525]
        n234 = for {
          N: w528 -> [_]
          tunnel: w527 -> [w540]
          shift-right: [w537] -> w529
          shift-left: w530 -> [w538]
          tunnel: w526 -> [w531]
          tunnel: w525 -> [w536]
          tunnel: w524 -> [w535]
          i -> [w539]
          n235 = Multiply(x=w540, y=w539) -> (x*y=w533:i32)
          n236 = Multiply(x=w535, y=w536) -> (x*y=w534:i32)
          n237 = Add(x=w533, y=w534) -> (x+y=w532:i32)
          n238 = Replace Array Subset(array=w538, new element=w531, index=w532) -> (w537:dbl[])
        }
      }
      n239 = Build Array (concatenate)(w465, w462) -> (w464:dbl[])
      n240 = Build Array (concatenate)(w474, w463) -> (w475:dbl[])
      n241 = Quotient & Remainder(x=w443, y=2) -> (x-y*floor(x/y)=w455:u32)  [unwired: 1 out]
      n242 = for {
        N: w443 -> [_]
        shift-right: [w509] -> w454
        shift-left: dbl[] [] -> [w510]
        tunnel: w475 -> [w511]
        tunnel: w464 -> [w508]
        i -> [w506]
        n243 = Quotient & Remainder(x=w506, y=2) -> (x-y*floor(x/y)=w507:i32)  [unwired: 1 out]
        n244 = case shown="0, Default" w507 {
          tunnel: w511 -> [w515 _]
          tunnel: w510 -> [w514 w517]
          tunnel: [w513 w516] -> w509
          tunnel: w508 -> [_ w518]
          frame 0, Default {
            n245 = Build Array (concatenate)(w514, w515) -> (w513:dbl[])
          }
          frame 1 {
            n246 = Build Array (concatenate)(w517, w518) -> (w516:dbl[])
          }
        }
      }
      n247 = Divide(x=w480, y=2.0) -> (x/y=w487:dbl)
      n248 = case shown="0, Default" w455 {
        tunnel: w458 -> [_ w500]
        tunnel: w457 -> [w499 _]
        tunnel: [w499 w500] -> w456
        frame 0, Default {
        }
        frame 1 {
        }
      }
      n249 = Add(x=w437, y=w487) -> (x+y=w486:dbl)
      n250 = Round Toward -Infinity(1:w486) -> (0:w485:dbl)
      n251 = To Word Integer(number=w485) -> (16bit integer=w484:i16)
      n252 = Initialize Array(w456, w461) -> (w453:dbl[])
      n253 = Initialize Array(u32 0 ("element"), w441) -> (w450:u32[])
      n254 = Build Array (concatenate)(w454, w453) -> (w451:dbl[])
      n255 = Rotate 1D Array(1:w477, 2:w484) -> (0:w476:dbl[])
    }
    frame 5 {
      # "Note (simplified version): \n1. if multi 3D, use mode 3\n2. n_frames must be divider of Rep"
      n256 = script code="t1=[5*ones(1,n_lines), zeros(1,flyback_lines)];\nt_data=repmat(t1,1,n_frames);\n\nx1=x_center+[linspace(-x_span/2,x_span/2,n_lines),x_span/2*cos(linspace(0,pi,flyback_lines))];\nx_data=repmat(x1,1,n_frames);\nx_data=circshift(x_data,[0,GalvoPhase]);\n\n%x1=[x_center+linspace(-x_span/2,x_span/2,n_lines),linspace(x_span/2,-x_span/2,flyback_lines)];\n%x_data=repmat(x1,1,n_frames);\n%x_data=circshift(x_data,[0,GalvoPhase]);\n\ny1=linspace(-y_span/2,y_span/2,n_frames/Rep);\ny_data=y_center+reshape(repmat(y1,Rep*Line,1),1,[]);"("n_lines"=w554, "n_frames"=w553, "flyback_lines"=w552, "y_center"=w551, "y_span"=w550, "x_center"=w549, "x_span"=w548, "GalvoPhase"=w547, "Rep"=w543, "Line"=w542) -> ("??"=w541:errorcluster, "t_data"=w546:dbl[], "x_data"=w545:dbl[], "y_data"=w544:dbl[])  [unwired: 1 in]
    }
    frame 25 {
      # "Note: \nThis mode is for Lei's Doppler Protocol."
      n257 = script code="XRep=4;\n\nt1=[zeros(1,50),5*ones(1,50),zeros(1,n_lines+flyback_lines-100)];\nt_data=repmat(t1,1,n_frames);\n\nxstep=reshape(repmat(linspace(-x_span/2,x_span/2,n_lines/XRep),[XRep,1]),[1,n_lines]);\nx1=x_center+[xstep,x_span/2*cos(linspace(0,pi,flyback_lines))];\nx_data=repmat(x1,1,n_frames);\nx_data=circshift(x_data,[0,GalvoPhase]);\n\n%x1=[x_center+linspace(-x_span/2,x_span/2,n_lines),linspace(x_span/2,-x_span/2,flyback_lines)];\n%x_data=repmat(x1,1,n_frames);\n%x_data=circshift(x_data,[0,GalvoPhase]);\n\ny1=linspace(-y_span/2,y_span/2,n_frames/Rep);\ny_data=y_center+reshape(repmat(y1,Rep*Line,1),1,[]);"("n_lines"=w568, "n_frames"=w567, "flyback_lines"=w566, "y_center"=w565, "y_span"=w564, "x_center"=w563, "x_span"=w562, "GalvoPhase"=w561, "Rep"=w557, "Line"=w556) -> ("??"=w555:errorcluster, "t_data"=w560:dbl[], "x_data"=w559:dbl[], "y_data"=w558:dbl[])  [unwired: 1 in]
    }
    frame 45 {
      # "Note: \nThis mode is for Shaozhen's Doppler Protocol.\nn_frames=number of positions. 160000\nn_lines=50\nnflyback_line=50\nRep=number of positions per B-scan."
      n258 = script code="% close all;\n% n_lines=25;  % M-mode repetition\n% flyback_lines=25;\n% Line=n_lines+flyback_lines;\n% n_frames=600;   %A-position*B-position, C-position=n_frames/Rep\n% x_span=8;y_span=8;\n% y_center=0;\n% Rep=300;    % A-position\n% GalvoPhase=0;  %should be 0 for Doppler. Don't be positive value\n\n%%\n\nt1=[zeros(1,flyback_lines),5,zeros(1,Line-flyback_lines-1)];\nt_data=repmat(t1,1,n_frames);\n\nx1=reshape(repmat(linspace(-x_span/2,x_span/2,Rep),[Line,1]),[1,Line*Rep]);\nx_data=repmat(x1,1,n_frames/Rep);\nx_data=circshift(x_data,[0,GalvoPhase]);\n\ny1=linspace(-y_span/2,y_span/2,n_frames/Rep);\ny_data=y_center+reshape(repmat(y1,Rep*Line,1),1,[]);\n\n%%\n% figure(1);\n% plot(x_data(:),'r');hold on;plot(y_data(:),'b');hold on;\n% plot(t_data,'g');"("n_lines"=w582, "n_frames"=w581, "flyback_lines"=w580, "y_center"=w579, "y_span"=w578, "x_center"=w577, "x_span"=w576, "GalvoPhase"=w575, "Rep"=w571, "Line"=w570) -> ("??"=w569:errorcluster, "t_data"=w574:dbl[], "x_data"=w573:dbl[], "y_data"=w572:dbl[])  [unwired: 1 in]
    }
    frame 35 {
      # "Note: \nThis mode is for Lei's Doppler Protocol."
      n259 = script code="ARep=1;\nBAppend=4;\n\nt1=[zeros(1,10),5*ones(1,10),zeros(1,Line-20)];\nt_data=repmat([repmat(t1,1,Rep),repmat(zeros(1,Line),1,BAppend)],1,n_frames/Rep);\n\nxstep=reshape(repmat(linspace(-x_span/2,x_span/2,n_lines/ARep),[ARep,1]),[1,n_lines]);\nx1=x_center+[xstep,x_span/2*cos(linspace(0,pi,flyback_lines))];\nx_data=repmat(x1,1,n_frames*(Rep+BAppend)/Rep);\nx_data=circshift(x_data,[0,GalvoPhase]);\n\n%x1=[x_center+linspace(-x_span/2,x_span/2,n_lines),linspace(x_span/2,-x_span/2,flyback_lines)];\n%x_data=repmat(x1,1,n_frames);\n%x_data=circshift(x_data,[0,GalvoPhase]);\n\ny1=linspace(-y_span/2,y_span/2,n_frames/Rep);\ny_data=y_center+reshape(repmat(y1,(Rep+BAppend)*Line,1),1,[]);"("n_lines"=w596, "n_frames"=w595, "flyback_lines"=w594, "y_center"=w593, "y_span"=w592, "x_center"=w591, "x_span"=w590, "GalvoPhase"=w589, "Rep"=w585, "Line"=w584) -> ("??"=w583:errorcluster, "t_data"=w588:dbl[], "x_data"=w587:dbl[], "y_data"=w586:dbl[])  [unwired: 1 in]
    }
    frame 6 {
      # "Note (simplified version): \n1. if multi 3D, use mode 3\n2. n_frames must be divider of Rep"
      n260 = script code="t1=[5*ones(1,n_lines), zeros(1,flyback_lines)];\nt_data=repmat(t1,1,n_frames);\n\nx1=[linspace(x_center-x_span/2,x_center+x_span/2,n_lines+floor(flyback_lines/4)),linspace(x_center+x_span/2,x_center-x_span/2,ceil(flyback_lines*3/4))];\nx_data=repmat(x1,1,n_frames);\nx_data=circshift(x_data,[0,GalvoPhase]);\n\ny1=linspace(-y_span/2,y_span/2,n_frames/n_3D/Rep);\ny_data1=y_center+reshape(repmat(y1,Rep*Line,1),1,[]);\ny_data=repmat(y_data1,1,n_3D);\ny_data=circshift(y_data,[0,GalvoPhase-ceil(flyback_lines*3/4)]);"("n_lines"=w600, "n_frames"=w598, "flyback_lines"=w597, "y_center"=w618, "y_span"=w617, "x_center"=w616, "x_span"=w615, "GalvoPhase"=w614, "Rep"=w610, "Line"=w609, "n_3D"=w608) -> ("??"=w607:errorcluster, "t_data"=w613:dbl[], "x_data"=w612:dbl[], "y_data"=w611:dbl[])  [unwired: 1 in]
      n261 = Initialize Array(u32 4294967295 ("new element/subarray"), w600) -> (w602:u32[])
      n262 = Initialize Array(u32 0 ("foo"), w597) -> (w601:u32[])
      n263 = Build Array (concatenate)(w602, w601) -> (w603:u32[])
      n264 = for {
        N: w598 -> [_]
        shift-right: [w620] -> w599
        shift-left: u32[] [] ("output array") -> [w621]
        tunnel: w603 -> [w619]
        n265 = Build Array (concatenate)(w621, w619) -> (w620:u32[])
      }
    }
    frame 9 {
      # "Note (simplified version): \n1. if multi 3D, use mode 3\n2. n_frames must be divider of Rep"
      n266 = script code="n_skip=1; % bidirection scan skip number\nnt=n_skip*2;\nnY=ceil((n_frames/n_3D/Rep)/nt)*nt;\n\nt1=[5*ones(1,n_lines), zeros(1,flyback_lines)];\nt_data=repmat(t1,1,n_frames);\n\nx1=[linspace(x_center-x_span/2,x_center+x_span/2,n_lines+flyback_lines),linspace(x_center+x_span/2,x_center-x_span/2,n_lines+flyback_lines)];\nx_data=repmat(x1,1,nY*Rep*n_3D/2);\nx_data=circshift(x_data,[0,GalvoPhase]);\n\n\ny1=linspace(-y_span/2,y_span/2,nY);\nn_group=nY/nt;\ny_tmp2=zeros(n_group,(n_lines+flyback_lines)*nt*Rep);\nfor i=1:n_group\n    y_tmp=reshape(repmat(y1((i-1)*nt+1:(i-1)*nt+nt),n_lines+flyback_lines,1),1,[]);\n    y_tmp2(i,:)=repmat(y_tmp,1,Rep);\nend\ny_tmp3=y_center+reshape(y_tmp2',1,[]);\ny_data=repmat(y_tmp3,1,n_3D);\ny_data=circshift(y_data,[0,GalvoPhase]);"("n_lines"=w625, "n_frames"=w622, "flyback_lines"=w624, "y_center"=w643, "y_span"=w642, "x_center"=w641, "x_span"=w640, "GalvoPhase"=w639, "Rep"=w635, "Line"=w634, "n_3D"=w633) -> ("??"=w632:errorcluster, "t_data"=w638:dbl[], "x_data"=w637:dbl[], "y_data"=w636:dbl[])  [unwired: 1 in]
      n267 = Initialize Array(u32 4294967295 ("new element/subarray"), w625) -> (w627:u32[])
      n268 = Initialize Array(u32 0 ("foo"), w624) -> (w626:u32[])
      n269 = Build Array (concatenate)(w627, w626) -> (w628:u32[])
      n270 = for {
        N: w622 -> [_]
        shift-right: [w645] -> w623
        shift-left: u32[] [] ("output array") -> [w646]
        tunnel: w628 -> [w644]
        n271 = Build Array (concatenate)(w646, w644) -> (w645:u32[])
      }
    }
    frame 7, Default {
      # "Note (simplified version): \n1. if multi 3D, use mode 3\n2. n_frames must be divider of Rep"
      n272 = script code="n_framesX = sqrt(n_frames); n_framesY = sqrt(n_frames);\nt1=[5*ones(1,n_lines),zeros(1,flyback_lines)];\nt_data=repmat(t1,1,n_framesX*n_framesY);\n\nx1=linspace(-x_span/2,x_span/2,n_framesX/n_3D/Rep);\nx_data1=x_center+reshape(repmat(x1,Rep*Line,1),1,[]);\nx_data=repmat(x_data1,1,n_3D);\n\nx_data=repmat(x_data,n_framesY,1);\nmask = ones(size(x_data));\nmask(2:2:n_framesY,:) = -1;\n\nx_data = x_data.*mask;\n% x_data(1:end-1,end-floor(flyback_lines*3/4):end) = x_data(2:end,1:floor(flyback_lines*3/4)+1);\nx_data = reshape(x_data',1,n_frames*Line);\nx_data=circshift(x_data,[0,GalvoPhase-floor(flyback_lines*3/4)]);\n\ny1=linspace(-y_span/2,y_span/2,n_framesY/n_3D/Rep);\ny_data1=y_center+reshape(repmat(y1,Rep*Line*n_framesX,1),1,[]);\ny_data=circshift(y_data1,[0,GalvoPhase-floor(flyback_lines*3/4)]);"("n_lines"=w649, "n_frames"=w648, "flyback_lines"=w650, "y_center"=w668, "y_span"=w667, "x_center"=w666, "x_span"=w665, "GalvoPhase"=w664, "Rep"=w662, "Line"=w661, "n_3D"=w657) -> ("??"=w658:errorcluster, "y_data"=w663:dbl[], "t_data"=w660:dbl[], "x_data"=w659:dbl[])  [unwired: 1 in]
      n273 = Initialize Array(u32 4294967295 ("new element/subarray"), w649) -> (w652:u32[])
      n274 = Initialize Array(u32 0 ("foo"), w650) -> (w651:u32[])
      n275 = Build Array (concatenate)(w652, w651) -> (w653:u32[])
      n276 = for {
        N: w648 -> [_]
        shift-right: [w670] -> w647
        shift-left: u32[] [] ("output array") -> [w671]
        tunnel: w653 -> [w669]
        n277 = Build Array (concatenate)(w671, w669) -> (w670:u32[])
      }
    }
    frame 8 {
      # "Note (simplified version): \n1. if multi 3D, use mode 3\n2. n_frames must be divider of Rep"
      n278 = script code="n_framesX = sqrt(n_frames); n_framesY = sqrt(n_frames);\nt1=[5*ones(1,n_lines),zeros(1,flyback_lines)];\nt_data=repmat(t1,1,n_framesX*n_framesY);\n\nx1=linspace(-x_span/2,x_span/2,n_framesX/n_3D/Rep);\nx_data1=x_center+reshape(repmat(x1,Rep*Line,1),1,[]);\nx_data=repmat(x_data1,1,n_3D);\nx_data=circshift(x_data,[0,GalvoPhase-ceil(flyback_lines*3/4)]);\nx_data=repmat(x_data,1,n_framesX);\n\ny1=linspace(-y_span/2,y_span/2,n_framesY/n_3D/Rep);\ny_data1=y_center+reshape(repmat(y1,Rep*Line*n_framesX,1),1,[]);\ny_data=circshift(y_data1,[0,GalvoPhase-ceil(flyback_lines*3/4)]);"("n_lines"=w686, "n_frames"=w685, "flyback_lines"=w684, "y_center"=w683, "y_span"=w682, "x_center"=w681, "x_span"=w680, "GalvoPhase"=w679, "Rep"=w677, "Line"=w676, "n_3D"=w675) -> ("??"=w672:errorcluster, "y_data"=w678:dbl[], "t_data"=w674:dbl[], "x_data"=w673:dbl[])  [unwired: 1 in]
    }
    frame 81 {
      # "Note (simplified version): \n1. if multi 3D, use mode 3\n2. n_frames must be divider of Rep"
      n279 = script code="if y_span>0\n   \n    nLperHalfGroup=n_lines*2*Rep+flyback_lines;\n    holdVector=ones(1,n_lines*2*Rep);\n    \n    nG=n_frames/4/Rep;\n    xG=linspace(-x_span/2,x_span/2,nG);\n    yG=linspace(-y_span/2,y_span/2,nG);\n    \n    x1=zeros(nLperHalfGroup*2,nG);\n    y1=zeros(nLperHalfGroup*2,nG);\n    \n    for iG=1:nG/2\n        x1(:,iG)=[repmat([xG,-xG],1,Rep),linspace(xG(iG),xG(iG),flyback_lines),xG(iG)*holdVector,linspace(xG(1),xG(1),flyback_lines)]';\n        y1(:,iG)=[yG(iG)*holdVector,linspace(yG(1),yG(1),flyback_lines),repmat([yG,-yG],1,Rep),linspace(yG(iG+1),yG(iG+1),flyback_lines)]';\n    end\n\n    x1(end-flyback_lines+1:end,iG)=-x1(end-flyback_lines+1:end,iG);\n\n    for iG=nG/2+1:nG-1\n        x1(:,iG)=[repmat([-xG,xG],1,Rep),linspace(xG(iG),xG(iG),flyback_lines),xG(iG)*holdVector,linspace(xG(end),xG(end),flyback_lines)]';\n        y1(:,iG)=[yG(iG)*holdVector,linspace(yG(end),yG(end),flyback_lines),repmat([-yG,yG],1,Rep),linspace(yG(iG+1),yG(iG+1),flyback_lines)]';\n    end\n    x1(:,nG)=[repmat([-xG,xG],1,Rep),linspace(xG(end),xG(nG),flyback_lines),xG(nG)*holdVector,linspace(xG(nG),xG(end),flyback_lines)]';\n    y1(:,nG)=[yG(nG)*holdVector,linspace(yG(nG),yG(end),flyback_lines),repmat([-yG,yG],1,Rep),linspace(yG(end),yG(nG),flyback_lines)]';\n    t1=zeros(1,nLperHalfGroup);\n    t1(1:n_lines:n_lines*2*Rep)=1;\n    t_data=repmat(t1,1,nG*2)*5;\nelse\n    nG=n_lines;\n    xG=linspace(-x_span/2,x_span/2,nG);\n    yG=linspace(-x_span/2,x_span/2,nG);\n    holdVector=ones(1,n_lines);\n    x1=[xG,linspace(xG(nG),0,flyback_lines),0*holdVector,linspace(0,xG(1),flyback_lines)];\n    y1=[0*holdVector,linspace(0,yG(1),flyback_lines),yG,linspace(yG(nG),0,flyback_lines)];\n    x1=repmat(x1,1,n_frames/2);\n    y1=repmat(y1,1,n_frames/2);\n    t1=zeros(1,(n_lines+flyback_lines)*2);\n    t1(1:(n_lines+flyback_lines):end)=1;\n    t_data=repmat(t1,1,n_frames/2)*5;\nend\n\nx_data=circshift(reshape(x1,1,[]),[0,GalvoPhase])+x_center; \ny_data=circshift(reshape(y1,1,[]),[0,GalvoPhase])+y_center;"("n_lines"=w706, "n_frames"=w705, "flyback_lines"=w704, "y_center"=w703, "y_span"=w702, "x_center"=w701, "x_span"=w700, "GalvoPhase"=w699, "Rep"=w697, "Line"=w696, "n_3D"=w695) -> ("??"=w693:errorcluster, "y_data"=w698:dbl[], "t_data"=w692:dbl[], "x_data"=w694:dbl[])  [unwired: 1 in]
      n280 = Divide(x=w692, y=5.0) -> (x/y=w688:dbl[])
      n281 = To Unsigned Long Integer(number=w688) -> (unsigned 32bit integer=w689:u32[])
      n282 = Multiply(x=w689, y=u32 4294967295 ("new element/subarray")) -> (x*y=w687:u32[])
    }
    frame 86 {
      # "Note (simplified version): \n1. if multi 3D, use mode 3\n2. n_frames must be divider of Rep"
      n283 = script code="if y_span>0\n    nLperGroup=n_lines*2*Rep+flyback_lines;\n    nG=n_frames/2/Rep;\n    xG=linspace(-x_span/2,x_span/2,n_lines);\n    yG=linspace(-y_span/2,y_span/2,nG);\n    yG(end+1)=yG(end);\n    \n    x1=zeros(nLperGroup,nG);\n    y1=zeros(nLperGroup,nG);\n    \n    for iG=1:nG\n        x1(:,iG)=[repmat([xG,-xG],1,Rep),ones(1,flyback_lines)*(-x_span/2)]';\n        y1(:,iG)=cat(1,yG(iG)*ones(n_lines*2*Rep,1),yG(iG+1)*ones(flyback_lines,1));\n    end\n    t1=zeros(1,nLperGroup);\n    t1(1:n_lines:n_lines*2*Rep)=1;\n    t_data=repmat(t1,1,nG)*5;\nelse\n    nG=n_lines;\n    xG=linspace(-x_span/2,x_span/2,nG);\n    yG=linspace(-x_span/2,x_span/2,nG);\n    holdVector=ones(1,n_lines);\n    x1=[xG,linspace(xG(nG),0,flyback_lines),0*holdVector,linspace(0,xG(1),flyback_lines)];\n    y1=[0*holdVector,linspace(0,yG(1),flyback_lines),yG,linspace(yG(nG),0,flyback_lines)];\n    x1=repmat(x1,1,n_frames/2);\n    y1=repmat(y1,1,n_frames/2);\n    t1=zeros(1,(n_lines+flyback_lines)*2);\n    t1(1:(n_lines+flyback_lines):end)=1;\n    t_data=repmat(t1,1,n_frames/2)*5;\nend\n\nx_data=circshift(reshape(x1,1,[]),[0,GalvoPhase])+x_center; \ny_data=circshift(reshape(y1,1,[]),[0,GalvoPhase])+y_center;"("n_lines"=w726, "n_frames"=w725, "flyback_lines"=w724, "y_center"=w723, "y_span"=w722, "x_center"=w721, "x_span"=w720, "GalvoPhase"=w719, "Rep"=w717, "Line"=w716, "n_3D"=w715) -> ("??"=w713:errorcluster, "y_data"=w718:dbl[], "t_data"=w708:dbl[], "x_data"=w714:dbl[])  [unwired: 1 in]
      n284 = Divide(x=w708, y=5.0) -> (x/y=w709:dbl[])
      n285 = To Unsigned Long Integer(number=w709) -> (unsigned 32bit integer=w710:u32[])
      n286 = Multiply(x=w710, y=u32 4294967295 ("new element/subarray")) -> (x*y=w707:u32[])
    }
    frame 36 {
      # "Note (simplified version): \n1. if multi 3D, use mode 3\n2. n_frames must be divider of Rep"
      n287 = script code="if y_span>0\n    t1=[5*ones(1,n_lines), zeros(1,flyback_lines)];\n    t_data=repmat(t1,1,n_frames);\n\n    x1=[linspace(x_center-x_span/2,x_center+x_span/2,n_lines+floor(flyback_lines/4)),linspace(x_center+x_span/2,x_center-x_span/2,ceil(flyback_lines*3/4))];\n    x_data=repmat(x1,1,n_frames);\n    x_data=circshift(x_data,[0,GalvoPhase]);\n\n    y1=linspace(-y_span/2,y_span/2,n_frames/n_3D/Rep);\n    y_data1=y_center+reshape(repmat(y1,Rep*Line,1),1,[]);\n    y_data=repmat(y_data1,1,n_3D);\n    y_data=circshift(y_data,[0,GalvoPhase-ceil(flyback_lines*3/4)]);\nelse\n    xG=linspace(-x_span/2,x_span/2,n_lines);\n    xGf=linspace(x_span/2,-x_span/2,flyback_lines);\n    yG=ones(1,n_lines);\n    yGf1=linspace(-x_span/2,0,flyback_lines);\n    yGf2=linspace(0,x_span/2,flyback_lines);\n    yGf3=linspace(x_span/2,-x_span/2,flyback_lines);\n    x1=repmat([xG,xGf],1,3);\n    y1=[-yG*x_span/2,yGf1,yG*0,yGf2,yG*x_span/2,yGf3];\n    t1=zeros(1,n_lines+flyback_lines);\n    t1(1)=1;\n    t_data=repmat(t1,1,3)*5;\n\n    x_data=circshift(reshape(x1,1,[]),[0,GalvoPhase])+x_center; \n    y_data=circshift(reshape(y1,1,[]),[0,GalvoPhase])+y_center; \nend"("n_lines"=w746, "n_frames"=w745, "flyback_lines"=w744, "y_center"=w743, "y_span"=w742, "x_center"=w741, "x_span"=w740, "GalvoPhase"=w739, "Rep"=w737, "Line"=w736, "n_3D"=w735) -> ("??"=w733:errorcluster, "y_data"=w738:dbl[], "t_data"=w728:dbl[], "x_data"=w734:dbl[])  [unwired: 1 in]
      n288 = Divide(x=w728, y=5.0) -> (x/y=w729:dbl[])
      n289 = To Unsigned Long Integer(number=w729) -> (unsigned 32bit integer=w730:u32[])
      n290 = Multiply(x=w730, y=u32 4294967295 ("new element/subarray")) -> (x*y=w727:u32[])
    }
    frame 15 {
      # "start"
      # "end"
      # "make sure that final array has size n_frames by appending right amount of elements at final y-pos."
      # "end"
      # "start"
      # "For resonant Galvo - Microangiography case, scan multiple frames at same y-position\n----------------------------\nslow axis gets one sample per frame\nno trig out and x-axis needed\nn_blank & start-doubleframes make no sense"
      n291 = Multiply(x=w770, y=0.5) -> (x*y=w772:dbl)
      n292 = Quotient & Remainder(x=w759, y=w747) -> (x-y*floor(x/y)=w758:u32, floor(x/y)=w755:u32)
      n293 = Subtract(x=w771, y=w772) -> (x-y=w753:dbl)
      n294 = Quotient & Remainder(x=w755, y=w766) -> (x-y*floor(x/y)=w748:u32, floor(x/y)=w762:u32)
      n295 = Add(x=w770, y=w753) -> (x+y=w754:dbl)
      n296 = Initialize Array(w754, w748) -> (w761:dbl[])
      n297 = Initialize Array(w753, w748) -> (w760:dbl[])
      n298 = call-poly <vilib>:"Ramp Pattern.vi"("start"=w753, "end"=w754, "samples"=w762) -> ("Ramp Pattern"=w776:dbl[])  [unwired: 7 in, 1 out]
      n299 = call-poly <vilib>:"Ramp Pattern.vi"("start"=w754, "end"=w753, "samples"=w762) -> ("Ramp Pattern"=w767:dbl[])  [unwired: 7 in, 1 out]
      n300 = for {
        tunnel: w776 -> [w805] mode=indexing
        tunnel: w766 -> [w802]
        shift-right: [w801] -> w779
        shift-left: dbl[] [] -> [w803]
        n301 = Initialize Array(w805, w802) -> (w804:dbl[])
        n302 = Build Array (concatenate)(w803, w804) -> (w801:dbl[])
      }
      n303 = for {
        tunnel: w767 -> [w787] mode=indexing
        tunnel: w766 -> [w784]
        shift-right: [w783] -> w764
        shift-left: dbl[] [] -> [w785]
        n304 = Initialize Array(w787, w784) -> (w786:dbl[])
        n305 = Build Array (concatenate)(w785, w786) -> (w783:dbl[])
      }
      n306 = Build Array (concatenate)(w764, w760) -> (w763:dbl[])
      n307 = Build Array (concatenate)(w779, w761) -> (w780:dbl[])
      n308 = Quotient & Remainder(x=w747, y=2) -> (x-y*floor(x/y)=w751:u32)  [unwired: 1 out]
      n309 = for {
        N: w747 -> [_]
        shift-right: [w791] -> w750
        shift-left: dbl[] [] -> [w792]
        tunnel: w780 -> [w793]
        tunnel: w763 -> [w790]
        i -> [w788]
        n310 = Quotient & Remainder(x=w788, y=2) -> (x-y*floor(x/y)=w789:i32)  [unwired: 1 out]
        n311 = case shown="1" w789 {
          tunnel: w793 -> [w797 _]
          tunnel: w792 -> [w796 w799]
          tunnel: [w795 w798] -> w791
          tunnel: w790 -> [_ w800]
          frame 0, Default {
            n312 = Build Array (concatenate)(w796, w797) -> (w795:dbl[])
          }
          frame 1 {
            n313 = Build Array (concatenate)(w799, w800) -> (w798:dbl[])
          }
        }
      }
      n314 = case shown="1" w751 {
        tunnel: w754 -> [_ w782]
        tunnel: w753 -> [w781 _]
        tunnel: [w781 w782] -> w752
        frame 0, Default {
        }
        frame 1 {
        }
      }
      n315 = Initialize Array(w752, w758) -> (w749:dbl[])
      n316 = Initialize Array(u32 0 ("element"), w759) -> (w769:u32[])
      n317 = Initialize Array(0.0 ("element"), w759) -> (w768:dbl[])
      n318 = Build Array (concatenate)(w750, w749) -> (w757:dbl[])
    }
    frame 16 {
      # "start"
      # "end"
      # "make sure that final array has size n_frames by appending right amount of elements at final y-pos."
      # "end"
      # "start"
      # "For resonant Galvo - Microangiography case, scan multiple frames at same y-position\n----------------------------\nslow axis gets one sample per frame\nno trig out and x-axis needed\nn_blank & start-doubleframes make no sense"
      n319 = Multiply(x=w840, y=0.5) -> (x*y=w842:dbl)
      n320 = Quotient & Remainder(x=w812, y=w820) -> (x-y*floor(x/y)=w830:u32, floor(x/y)=w827:u32)
      n321 = Subtract(x=w841, y=w842) -> (x-y=w826:dbl)
      n322 = Quotient & Remainder(x=w827, y=w837) -> (x-y*floor(x/y)=w821:u32, floor(x/y)=w833:u32)
      n323 = Initialize Array(0.0 ("element"), w819) -> (w815:dbl[])
      n324 = Add(x=w840, y=w826) -> (x+y=w806:dbl)
      n325 = for {
        N: w818 -> [_]
        tunnel: w817 -> [w858]
        tunnel: w816 -> [w857]
        shift-right: [w853] -> w814
        shift-left: dbl[] [] -> [w852]
        n326 = Initialize Array(5.0 ("element"), w858) -> (w856:dbl[])
        n327 = Initialize Array(0.0 ("element"), w857) -> (w854:dbl[])
        n328 = Build Array (concatenate)(w852, w856, w854) -> (w853:dbl[])
      }
      n329 = Initialize Array(w806, w821) -> (w832:dbl[])
      n330 = Initialize Array(w826, w821) -> (w831:dbl[])
      n331 = call-poly <vilib>:"Ramp Pattern.vi"("start"=w826, "end"=w806, "samples"=w833) -> ("Ramp Pattern"=w846:dbl[])  [unwired: 7 in, 1 out]
      n332 = call-poly <vilib>:"Ramp Pattern.vi"("start"=w806, "end"=w826, "samples"=w833) -> ("Ramp Pattern"=w838:dbl[])  [unwired: 7 in, 1 out]
      n333 = for {
        tunnel: w846 -> [w883] mode=indexing
        tunnel: w837 -> [w880]
        shift-right: [w879] -> w849
        shift-left: dbl[] [] -> [w881]
        n334 = Initialize Array(w883, w880) -> (w882:dbl[])
        n335 = Build Array (concatenate)(w881, w882) -> (w879:dbl[])
      }
      n336 = for {
        tunnel: w838 -> [w865] mode=indexing
        tunnel: w837 -> [w862]
        shift-right: [w861] -> w835
        shift-left: dbl[] [] -> [w863]
        n337 = Initialize Array(w865, w862) -> (w864:dbl[])
        n338 = Build Array (concatenate)(w863, w864) -> (w861:dbl[])
      }
      n339 = Build Array (concatenate)(w815, w814) -> (w810:dbl[])
      n340 = Build Array (concatenate)(w835, w831) -> (w834:dbl[])
      n341 = Build Array (concatenate)(w849, w832) -> (w850:dbl[])
      n342 = Quotient & Remainder(x=w820, y=2) -> (x-y*floor(x/y)=w824:u32)  [unwired: 1 out]
      n343 = Initialize Array(0.0 ("new element/subarray"), w812) -> (w809:dbl[])
      n344 = for {
        N: w820 -> [_]
        shift-right: [w869] -> w823
        shift-left: dbl[] [] -> [w870]
        tunnel: w850 -> [w871]
        tunnel: w834 -> [w868]
        i -> [w866]
        n345 = Quotient & Remainder(x=w866, y=2) -> (x-y*floor(x/y)=w867:i32)  [unwired: 1 out]
        n346 = case shown="1" w867 {
          tunnel: w871 -> [w875 _]
          tunnel: w870 -> [w874 w877]
          tunnel: [w873 w876] -> w869
          tunnel: w868 -> [_ w878]
          frame 0, Default {
            n347 = Build Array (concatenate)(w874, w875) -> (w873:dbl[])
          }
          frame 1 {
            n348 = Build Array (concatenate)(w877, w878) -> (w876:dbl[])
          }
        }
      }
      n349 = Replace Array Subset(array=w809, new element=w810, index=0) -> (w811:dbl[])
      n350 = case shown="1" w824 {
        tunnel: w806 -> [_ w860]
        tunnel: w826 -> [w859 _]
        tunnel: [w859 w860] -> w825
        frame 0, Default {
        }
        frame 1 {
        }
      }
      n351 = Initialize Array(w825, w830) -> (w822:dbl[])
      n352 = Initialize Array(u32 0 ("element"), w812) -> (w839:u32[])
      n353 = Build Array (concatenate)(w823, w822) -> (w829:dbl[])
    }
  }
  "x_data" <- w17
  "y_data" <- w20
  "trigger out" <- w41
  "t_data" <- w7
  n354 = Initialize Array(u32 0 ("new element/subarray"), w1) -> (w35:u32[])
  n355 = Initialize Array(u32 0 ("new element/subarray"), w37) -> (w36:u32[])
  n356 = Initialize Array(u32 4294967295 ("new element/subarray"), w1) -> (w29:u32[])
  n357 = for {
    N: w10 -> [_]
    shift-right: [w885] -> w27
    shift-left: w28 -> [w886]
    tunnel: w29 -> [w884]
    n358 = Build Array (concatenate)(w886, w884) -> (w885:u32[])
  }
  n359 = for {
    N: w12 -> [_]
    shift-right: [w888] -> w43
    shift-left: w28 -> [w889]
    tunnel: w35 -> [w887]
    n360 = Build Array (concatenate)(w889, w887) -> (w888:u32[])
  }
  n361 = Build Array (concatenate)(w27, w36) -> (w42:u32[])
  n362 = for {
    N: w13 -> [_]
    shift-right: [w890] -> w38
    shift-left: u32[] [] ("output array") -> [w892]
    tunnel: w42 -> [w891]
    n363 = Build Array (concatenate)(w892, w891) -> (w890:u32[])
  }
  n364 = Build Array (concatenate)(w43, w38) -> (w39:u32[])
  n365 = Array Size(array=w41) -> (size(s)=w31:i32)
  n366 = Array Size(array=w39) -> (size(s)=w40:i32)
  n367 = Subtract(x=w31, y=w40) -> (x-y=w32:i32)
  n368 = Greater Or Equal To 0?(x=w32) -> (x >= 0?=w33:bool)
  n369 = call <vilib>:"Simple Error Handler.vi"("error in (no error)"=w5) -> ()  [unwired: 4 in, 5 out]
  n370 = case shown="True" w33 {
    tunnel: w39 -> [w895 w899]
    tunnel: w32 -> [_ w898]
    tunnel: [w893 w896] -> w14
    tunnel: w31 -> [w894 _]
    frame False {
      n371 = Array Subset(array=w895, length=w894) -> (w893:u32[])  [unwired: 1 in]
    }
    frame True {
      n372 = Initialize Array(u32 0 ("foo"), w898) -> (w897:u32[])
      n373 = Build Array (concatenate)(w899, w897) -> (w896:u32[])
    }
  }
  "custom trig out" <- w14
  n374 = Array Size(array=w17) -> (size(s)=→"size(s)":i32)
